vi "Host-Scannig-Probe-Microscope-Controller-2014-12-05-RFR-version-for-MCL-drift-trial-fm-NanoH50-1b.vi"() -> ()   [LabVIEW 2012]
uses:
  <vilib>/FPGAPlugInAG/PCIe-7852R/niLvFpga_Open_PCIe-7852R.vi
  <vilib>/Utility/error.llb/Error Cluster From Error Code.vi
  <vilib>/rvi/errors/niLvFpgaAdjustHostInterfaceError.vi
  <vilib>/FPGAPlugInAG/PCIe-7852R/niLvFpga_Close_PCIe-7852R.vi
  <vilib>/FPGAPlugInAG/PCIe-7852R/niLvFpga_Run_PCIe-7852R.vi
  <vilib>/Utility/file.llb/Write To Spreadsheet File (I64).vi
  <vilib>/rvi/interface/nirviOpenFPGA/nirviOpenFPGA.xnode
  FPGA Bitfiles/2012-10-30-PhD_FPGATarget_Scannig-Probe-Mi_wQHWF7AZtyE.lvbitx
  Scannig-Probe-Microscope-Controller-2010-03-08-RFR-version-for-MCL-nanoh50-1b.vi
  <vilib>/rvi/interface/nirviMethod/nirviMethod.xnode
  <vilib>/rvi/interface/nirviReadWriteControl/nirviReadWriteControl.xnode
  <vilib>/rvi/interface/nirviCloseFPGA/nirviCloseFPGA.xnode
  <vilib>/rvi/errors/niLvFpgaMergeErrorWithErrorCode.vi
  <vilib>/FPGAPlugInAG/PCIe-7852R/niLvFpga_ReadFifo_PCIe-7852R.vi
  NiFpgaLv.dll
panel:
  out "fpga y images":i32
  out "hi(x)":u16[](array[numeric])=[32260, 32260, 32276, 32269, 32267, 32261, 32276, 32257, 32271, 32261, 32259, 32255, 32261, 32255, 32257, 32259, 32264, 32267, 32261, 32276, 32252, 32274, 32264, 32263, 32267, 32260, 32257, 32262, 32260, 32263, 32265, 32252, 32248, 32257, 32271, 32258, 32258, 32267, 32259, 32260, 32276, 32276, 32254, 32257, 32255, 32263, 32266, 32260, 32264, 32256, 32262, 32259, 32264, 32267, 32255, 32256, 32271, 32257, 32260, 32265, 32260, 32258, 32277, 32257, 32267, 32253, 32260, 32257, 32262, 32264, 32264, 32263, 32260, 32266, 32254, 32263, 32261, 32256, 32269, 32265, 32263, 32279, 32265, 32262, 32253, 32269, 32266, 32269, 32257, 32262, 32249, 32260, 32251, 32259, 32265, 32264, 32262, 32261, 32259, 32268, 32260, 32260, 32277, 32271, 32242, 32256, 32253, 32257, 32257, 32237, 32263, 32250, 32261, 32264, 32273, 32263, 32258, 32264, 32259, 32265, 32256, 32263, 32264, 32277, 32271, 32255, 32258, 32261]
  out "Y line":i32=1
  out "Time per step (us) /X axis sub pixels":u32=203
  in  "X axis pixels":u16=256
  in  "Lines per second":dbl=0.2 min=1e-05 max=50.0
  in  "Time per step/ Y axis sub pixels (usec)":u32=1200
  in  "X Size (um)":dbl=60.0
  in  "X Total Range (um)":dbl=80.0
  in  "Y Size (um)":dbl=60.0
  in  "Y Total Range (um)":dbl=80.0
  in  "Y axis pixels":u16=256
  in  "Timeout FIFO":i32=-1
  in  "x initial":i16
  in  "y initial":i16
  out "X axis steps per pixel":u16=96
  in  "Number of images":u32=10000
  out "Y axis steps per pixel":u16=96
  out "Pixels for one image":i32=131072
  in  "Internal Setpoint":i16=7166
  in  "I scale":i8=-8
  in  "P scale":i8=-2
  in  "Setpoint Control":bool=TRUE
  in  "PID gains (x 2^8)":T1={"proportional gain (Kc)"=1, "integral gain (Kc*Ts/Ti)"=11, "derivative gain (Kc*Td/Ts)"=0}
  in  "Forth/Back X axis":bool
  in  "Forth/Back Y axis":bool
  in  "Feedback loop time(uSec)":u8
  in  "Stop Feedback":bool=TRUE
  in  "Scanning On/Off":bool
  in  "offset retraction drift":i16
  in  "control for drift correction":u32=512000
  in  "time before averaging drift":u32=9000
  in  "drift averager":u16=100
  in  "drift Waiting (uSec)":u16=10
  in  "offset FM":u16=1000
  out "Steps Per Feedback region":u16=642
  in  "Number of Feedback Regions":u32=102
  in  "shift integrator control":i32=2000
  in  "upper limit regions":i16=99
  out "line shift":i32
  out "line in matrix":i32=254
  out "Y Output Value":i16
  out "image indicator":i32=1
  out "Bottom Sensor Magnitude Image":i16[][](graph)
  out "Trace Bottom Sensor Magnitude":i16[][](graph)=[[12, 13, 14, 14, 14, 14, 14, 14, 14, 14, 14, 14, 14, 14, 14, 14, 14, 14, 14, 14, 14, 14, 14, 14, 14, 14, 14, 14, 14, 14, 14, 14, 14, 14, 14, 14, 14, 14, 14, 14, 14, 14, 14, 14, 14, 14, 14, 14, 14, 14, 14, 14, 14, 14, 14, 14, 14, 14, 14, 14, 14, 14, 14, 14, 14, 14, 14, 14, 14, 14, 14, 14, 14, 14, 14, 14, 14, 14, 14, 14, 14, 14, 14, 14, 14, 14, 14, 14, 14, 14, 14, 14, 14, 14, 14, 14, 14, 14, 14, 14, 14, 14, 14, 14, 14, 14, 14, 14, 14, 14, 14, 14, 14, 14, 14, 14, 14, 14, 14, 14, 14, 14, 14, 14, 14, 14, 14, 14, 14, 14, 14, 14, 14, 14, 14, 14, 14, 14, 14, 14, 14, 14, 14, 14, 14, 14, 14, 14, 14, 14, 14, 14, 14, 14, 14, 14, 14, 14, 14, 14, 14, 14, 14, 14, 14, 14, 14, 14, 14, 14, 14, 14, 14, 14, 14, 14, 14, 14, 14, 14, 14, 14, 14, 14, 14, 14, 14, 14, 14, 14, 14, 14, 14, 14, 14, 14, 14, 14, 14, 14, 14, 14, 14, 14, 14, 14, 14, 14, 14, 14, 14, 14, 14, 14, 14, 14, 14, 14, 14, 14, 14, 14, 14, 14, 14, 14, 14, 14, 14, 14, 14, 14, 14, 14, 14, 14, 14, 14, 14, 14, 14, 14, 14, 14, 14, 14, 14, 14, 14, 14, 14, 14, 14, 14, 14, 14], [10, 10, 10, 10, 11, 11, 11, 10, 10, 10, 10, 10, 10, 10, 10, 10, 10, 10, 10, 10, 10, 10, 10, 11, 11, 10, 10, 11, 11, 11, 11, 10, 10, 10, 10, 10, 10, 10, 10, 10, 11, 11, 10, 10, 11, 11, 11, 11, 11, 11, 10, 11, 11, 11, 11, 10, 10, 10, 10, 11, 10, 10, 10, 10, 10, 10, 10, 10, 10, 10, 11, 10, 10, 10, 10, 11, 11, 10, 10, 10, 10, 10, 10, 10, 10, 10, 10, 10, 10, 10, 10, 10, 10, 10, 10, 10, 10, 10, 10, 10, 10, 10, 10, 10, 10, 10, 10, 10, 10, 10, 11, 11, 10, 10, 10, 10, 11, 11, 11, 10, 10, 11, 10, 10, 10, 11, 11, 11, 11, 10, 10, 11, 11, 11, 10, 10, 11, 11, 10, 10, 10, 10, 10, 10, 10, 10, 11, 10, 10, 10, 10, 11, 11, 10, 10, 10, 10, 10, 10, 11, 11, 11, 11, 11, 11, 10, 10, 10, 10, 10, 10, 10, 10, 10, 10, 10, 10, 10, 10, 10, 10, 10, 10, 10, 11, 11, 10, 10, 10, 10, 10, 10, 11, 10, 10, 10, 11, 10, 10, 10, 10, 10, 10, 10, 10, 10, 10, 11, 11, 10, 10, 10, 11, 10, 10, 10, 10, 10, 10, 10, 10, 10, 11, 10, 10, 10, 10, 11, 11, 10, 10, 11, 11, 11, 11, 11, 11, 10, 10, 11, 11, 11, 11, 11, 11, 10, 10, 10, 10, 11, 10, 10, 10, 11, 13, 14]]
  out "TF Magnitude Image":i16[][](graph)
  out "Trace TF Magnitud":i16[][](graph)=[[18, 18, 18, 18, 18, 18, 18, 19, 19, 17, 17, 17, 18, 18, 18, 18, 18, 18, 18, 18, 18, 18, 18, 17, 17, 17, 17, 18, 18, 18, 17, 16, 16, 16, 16, 17, 18, 19, 20, 20, 19, 18, 18, 18, 18, 18, 18, 18, 17, 16, 16, 18, 19, 19, 18, 18, 18, 19, 20, 19, 18, 18, 18, 18, 18, 18, 18, 18, 18, 18, 17, 17, 17, 18, 18, 18, 18, 18, 18, 17, 17, 17, 18, 18, 18, 17, 16, 17, 17, 17, 17, 18, 18, 18, 17, 17, 18, 17, 17, 17, 17, 18, 18, 18, 18, 18, 18, 18, 17, 17, 18, 18, 18, 18, 18, 18, 18, 18, 19, 20, 19, 18, 16, 17, 18, 18, 17, 17, 17, 18, 18, 17, 17, 17, 16, 17, 18, 18, 18, 18, 18, 18, 18, 18, 17, 17, 17, 16, 16, 17, 18, 18, 18, 17, 17, 18, 19, 19, 18, 18, 18, 18, 17, 17, 18, 18, 18, 17, 17, 17, 17, 18, 18, 18, 18, 18, 17, 17, 17, 17, 17, 18, 18, 18, 18, 18, 18, 18, 18, 18, 18, 17, 16, 17, 17, 18, 19, 20, 19, 18, 18, 18, 18, 18, 17, 16, 16, 16, 16, 16, 16, 17, 18, 18, 17, 16, 17, 18, 18, 18, 18, 18, 17, 18, 18, 18, 18, 18, 18, 17, 17, 18, 18, 18, 18, 18, 18, 18, 18, 18, 19, 20, 19, 19, 18, 18, 18, 18, 17, 17, 17, 17, 18, 18, 18, 17], [17, 17, 17, 17, 17, 18, 18, 18, 18, 18, 18, 18, 17, 17, 17, 18, 18, 18, 19, 19, 19, 18, 18, 17, 18, 18, 18, 18, 18, 17, 18, 18, 19, 19, 18, 17, 17, 17, 17, 17, 17, 17, 17, 17, 17, 18, 18, 17, 17, 18, 19, 18, 17, 18, 18, 18, 18, 17, 17, 17, 18, 18, 18, 17, 16, 16, 17, 18, 19, 19, 18, 18, 19, 19, 18, 18, 18, 18, 17, 17, 16, 17, 18, 18, 18, 18, 18, 17, 17, 17, 18, 18, 18, 19, 18, 18, 17, 17, 17, 16, 16, 17, 16, 17, 18, 18, 18, 18, 18, 18, 18, 18, 18, 18, 18, 19, 20, 20, 19, 18, 18, 18, 18, 18, 19, 19, 18, 17, 17, 18, 18, 18, 18, 18, 18, 17, 18, 18, 18, 18, 17, 17, 17, 17, 18, 18, 18, 18, 18, 18, 17, 17, 17, 18, 18, 18, 18, 18, 18, 18, 18, 18, 18, 18, 18, 18, 18, 17, 17, 18, 18, 18, 18, 18, 18, 18, 18, 18, 18, 18, 18, 18, 18, 18, 17, 17, 18, 18, 18, 18, 17, 17, 17, 18, 18, 18, 18, 18, 18, 18, 18, 18, 18, 18, 18, 17, 16, 16, 16, 17, 18, 18, 18, 18, 17, 17, 17, 18, 18, 18, 17, 16, 17, 18, 18, 18, 18, 18, 18, 18, 18, 17, 16, 17, 18, 18, 18, 18, 18, 18, 18, 18, 18, 18, 18, 18, 18, 18, 17, 17, 18, 18, 18, 18, 18, 17]]
  out "Trace AI5 array":i16[][](array[numeric])=[[12, 13, 14, 14, 14, 14, 14, 14, 14, 14, 14, 14, 14, 14, 14, 14, 14, 14, 14, 14, 14, 14, 14, 14, 14, 14, 14, 14, 14, 14, 14, 14, 14, 14, 14, 14, 14, 14, 14, 14, 14, 14, 14, 14, 14, 14, 14, 14, 14, 14, 14, 14, 14, 14, 14, 14, 14, 14, 14, 14, 14, 14, 14, 14, 14, 14, 14, 14, 14, 14, 14, 14, 14, 14, 14, 14, 14, 14, 14, 14, 14, 14, 14, 14, 14, 14, 14, 14, 14, 14, 14, 14, 14, 14, 14, 14, 14, 14, 14, 14, 14, 14, 14, 14, 14, 14, 14, 14, 14, 14, 14, 14, 14, 14, 14, 14, 14, 14, 14, 14, 14, 14, 14, 14, 14, 14, 14, 14, 14, 14, 14, 14, 14, 14, 14, 14, 14, 14, 14, 14, 14, 14, 14, 14, 14, 14, 14, 14, 14, 14, 14, 14, 14, 14, 14, 14, 14, 14, 14, 14, 14, 14, 14, 14, 14, 14, 14, 14, 14, 14, 14, 14, 14, 14, 14, 14, 14, 14, 14, 14, 14, 14, 14, 14, 14, 14, 14, 14, 14, 14, 14, 14, 14, 14, 14, 14, 14, 14, 14, 14, 14, 14, 14, 14, 14, 14, 14, 14, 14, 14, 14, 14, 14, 14, 14, 14, 14, 14, 14, 14, 14, 14, 14, 14, 14, 14, 14, 14, 14, 14, 14, 14, 14, 14, 14, 14, 14, 14, 14, 14, 14, 14, 14, 14, 14, 14, 14, 14, 14, 14, 14, 14, 14, 14, 14, 14], [10, 10, 10, 10, 11, 11, 11, 10, 10, 10, 10, 10, 10, 10, 10, 10, 10, 10, 10, 10, 10, 10, 10, 11, 11, 10, 10, 11, 11, 11, 11, 10, 10, 10, 10, 10, 10, 10, 10, 10, 11, 11, 10, 10, 11, 11, 11, 11, 11, 11, 10, 11, 11, 11, 11, 10, 10, 10, 10, 11, 10, 10, 10, 10, 10, 10, 10, 10, 10, 10, 11, 10, 10, 10, 10, 11, 11, 10, 10, 10, 10, 10, 10, 10, 10, 10, 10, 10, 10, 10, 10, 10, 10, 10, 10, 10, 10, 10, 10, 10, 10, 10, 10, 10, 10, 10, 10, 10, 10, 10, 11, 11, 10, 10, 10, 10, 11, 11, 11, 10, 10, 11, 10, 10, 10, 11, 11, 11, 11, 10, 10, 11, 11, 11, 10, 10, 11, 11, 10, 10, 10, 10, 10, 10, 10, 10, 11, 10, 10, 10, 10, 11, 11, 10, 10, 10, 10, 10, 10, 11, 11, 11, 11, 11, 11, 10, 10, 10, 10, 10, 10, 10, 10, 10, 10, 10, 10, 10, 10, 10, 10, 10, 10, 10, 11, 11, 10, 10, 10, 10, 10, 10, 11, 10, 10, 10, 11, 10, 10, 10, 10, 10, 10, 10, 10, 10, 10, 11, 11, 10, 10, 10, 11, 10, 10, 10, 10, 10, 10, 10, 10, 10, 11, 10, 10, 10, 10, 11, 11, 10, 10, 11, 11, 11, 11, 11, 11, 10, 10, 11, 11, 11, 11, 11, 11, 10, 10, 10, 10, 11, 10, 10, 10, 11, 13, 14]]
  out "Trace AI5 temp":i16[](array[numeric])=[12, 13, 14, 14, 14, 14, 14, 14, 14, 14, 14, 14, 14, 14, 14, 14, 14, 14, 14, 14, 14, 14, 14, 14, 14, 14, 14, 14, 14, 14, 14, 14, 14, 14, 14, 14, 14, 14, 14, 14, 14, 14, 14, 14, 14, 14, 14, 14, 14, 14, 14, 14, 14, 14, 14, 14, 14, 14, 14, 14, 14, 14, 14, 14, 14, 14, 14, 14, 14, 14, 14, 14, 14, 14, 14, 14, 14, 14, 14, 14, 14, 14, 14, 14, 14, 14, 14, 14, 14, 14, 14, 14, 14, 14, 14, 14, 14, 14, 14, 14, 14, 14, 14, 14, 14, 14, 14, 14, 14, 14, 14, 14, 14, 14, 14, 14, 14, 14, 14, 14, 14, 14, 14, 14, 14, 14, 14, 14, 14, 14, 14, 14, 14, 14, 14, 14, 14, 14, 14, 14, 14, 14, 14, 14, 14, 14, 14, 14, 14, 14, 14, 14, 14, 14, 14, 14, 14, 14, 14, 14, 14, 14, 14, 14, 14, 14, 14, 14, 14, 14, 14, 14, 14, 14, 14, 14, 14, 14, 14, 14, 14, 14, 14, 14, 14, 14, 14, 14, 14, 14, 14, 14, 14, 14, 14, 14, 14, 14, 14, 14, 14, 14, 14, 14, 14, 14, 14, 14, 14, 14, 14, 14, 14, 14, 14, 14, 14, 14, 14, 14, 14, 14, 14, 14, 14, 14, 14, 14, 14, 14, 14, 14, 14, 14, 14, 14, 14, 14, 14, 14, 14, 14, 14, 14, 14, 14, 14, 14, 14, 14, 14, 14, 14, 14, 14, 14]
  out "Trace AI6  array":i16[][](array[numeric])=[[18, 18, 18, 18, 18, 18, 18, 19, 19, 17, 17, 17, 18, 18, 18, 18, 18, 18, 18, 18, 18, 18, 18, 17, 17, 17, 17, 18, 18, 18, 17, 16, 16, 16, 16, 17, 18, 19, 20, 20, 19, 18, 18, 18, 18, 18, 18, 18, 17, 16, 16, 18, 19, 19, 18, 18, 18, 19, 20, 19, 18, 18, 18, 18, 18, 18, 18, 18, 18, 18, 17, 17, 17, 18, 18, 18, 18, 18, 18, 17, 17, 17, 18, 18, 18, 17, 16, 17, 17, 17, 17, 18, 18, 18, 17, 17, 18, 17, 17, 17, 17, 18, 18, 18, 18, 18, 18, 18, 17, 17, 18, 18, 18, 18, 18, 18, 18, 18, 19, 20, 19, 18, 16, 17, 18, 18, 17, 17, 17, 18, 18, 17, 17, 17, 16, 17, 18, 18, 18, 18, 18, 18, 18, 18, 17, 17, 17, 16, 16, 17, 18, 18, 18, 17, 17, 18, 19, 19, 18, 18, 18, 18, 17, 17, 18, 18, 18, 17, 17, 17, 17, 18, 18, 18, 18, 18, 17, 17, 17, 17, 17, 18, 18, 18, 18, 18, 18, 18, 18, 18, 18, 17, 16, 17, 17, 18, 19, 20, 19, 18, 18, 18, 18, 18, 17, 16, 16, 16, 16, 16, 16, 17, 18, 18, 17, 16, 17, 18, 18, 18, 18, 18, 17, 18, 18, 18, 18, 18, 18, 17, 17, 18, 18, 18, 18, 18, 18, 18, 18, 18, 19, 20, 19, 19, 18, 18, 18, 18, 17, 17, 17, 17, 18, 18, 18, 17], [17, 17, 17, 17, 17, 18, 18, 18, 18, 18, 18, 18, 17, 17, 17, 18, 18, 18, 19, 19, 19, 18, 18, 17, 18, 18, 18, 18, 18, 17, 18, 18, 19, 19, 18, 17, 17, 17, 17, 17, 17, 17, 17, 17, 17, 18, 18, 17, 17, 18, 19, 18, 17, 18, 18, 18, 18, 17, 17, 17, 18, 18, 18, 17, 16, 16, 17, 18, 19, 19, 18, 18, 19, 19, 18, 18, 18, 18, 17, 17, 16, 17, 18, 18, 18, 18, 18, 17, 17, 17, 18, 18, 18, 19, 18, 18, 17, 17, 17, 16, 16, 17, 16, 17, 18, 18, 18, 18, 18, 18, 18, 18, 18, 18, 18, 19, 20, 20, 19, 18, 18, 18, 18, 18, 19, 19, 18, 17, 17, 18, 18, 18, 18, 18, 18, 17, 18, 18, 18, 18, 17, 17, 17, 17, 18, 18, 18, 18, 18, 18, 17, 17, 17, 18, 18, 18, 18, 18, 18, 18, 18, 18, 18, 18, 18, 18, 18, 17, 17, 18, 18, 18, 18, 18, 18, 18, 18, 18, 18, 18, 18, 18, 18, 18, 17, 17, 18, 18, 18, 18, 17, 17, 17, 18, 18, 18, 18, 18, 18, 18, 18, 18, 18, 18, 18, 17, 16, 16, 16, 17, 18, 18, 18, 18, 17, 17, 17, 18, 18, 18, 17, 16, 17, 18, 18, 18, 18, 18, 18, 18, 18, 17, 16, 17, 18, 18, 18, 18, 18, 18, 18, 18, 18, 18, 18, 18, 18, 18, 17, 17, 18, 18, 18, 18, 18, 17]]
  out "TraceAI6 temp":i16[](array[numeric])=[18, 18, 18, 18, 18, 18, 18, 19, 19, 17, 17, 17, 18, 18, 18, 18, 18, 18, 18, 18, 18, 18, 18, 17, 17, 17, 17, 18, 18, 18, 17, 16, 16, 16, 16, 17, 18, 19, 20, 20, 19, 18, 18, 18, 18, 18, 18, 18, 17, 16, 16, 18, 19, 19, 18, 18, 18, 19, 20, 19, 18, 18, 18, 18, 18, 18, 18, 18, 18, 18, 17, 17, 17, 18, 18, 18, 18, 18, 18, 17, 17, 17, 18, 18, 18, 17, 16, 17, 17, 17, 17, 18, 18, 18, 17, 17, 18, 17, 17, 17, 17, 18, 18, 18, 18, 18, 18, 18, 17, 17, 18, 18, 18, 18, 18, 18, 18, 18, 19, 20, 19, 18, 16, 17, 18, 18, 17, 17, 17, 18, 18, 17, 17, 17, 16, 17, 18, 18, 18, 18, 18, 18, 18, 18, 17, 17, 17, 16, 16, 17, 18, 18, 18, 17, 17, 18, 19, 19, 18, 18, 18, 18, 17, 17, 18, 18, 18, 17, 17, 17, 17, 18, 18, 18, 18, 18, 17, 17, 17, 17, 17, 18, 18, 18, 18, 18, 18, 18, 18, 18, 18, 17, 16, 17, 17, 18, 19, 20, 19, 18, 18, 18, 18, 18, 17, 16, 16, 16, 16, 16, 16, 17, 18, 18, 17, 16, 17, 18, 18, 18, 18, 18, 17, 18, 18, 18, 18, 18, 18, 17, 17, 18, 18, 18, 18, 18, 18, 18, 18, 18, 19, 20, 19, 19, 18, 18, 18, 18, 17, 17, 17, 17, 18, 18, 18, 17]
  out "AI5 Back":i16[][](array[numeric])
  out "AI5 Array":i16[][](array[numeric])
  out "AI6 Array Back":i16[][](array[numeric])
  out "AI6 Array":i16[][](array[numeric])
  out "Internal Setpoint indicator":i16=7166
  out "iterations x":i32=1023
  out "Trace AI2 array":i16[][](array[numeric])=[[32261, 32262, 32263, 32251, 32270, 32257, 32263, 32257, 32274, 32262, 32258, 32261, 32254, 32263, 32267, 32265, 32263, 32260, 32249, 32260, 32251, 32264, 32255, 32260, 32266, 32263, 32269, 32248, 32264, 32262, 32268, 32250, 32269, 32263, 32260, 32264, 32263, 32260, 32236, 32261, 32253, 32255, 32266, 32261, 32263, 32258, 32276, 32246, 32255, 32242, 32251, 32252, 32264, 32263, 32258, 32254, 32261, 32247, 32260, 32251, 32249, 32263, 32256, 32251, 32273, 32242, 32249, 32257, 32259, 32262, 32260, 32251, 32264, 32260, 32267, 32257, 32267, 32257, 32270, 32255, 32253, 32261, 32258, 32264, 32261, 32261, 32259, 32266, 32261, 32255, 32254, 32243, 32258, 32270, 32261, 32268, 32265, 32260, 32259, 32262, 32263, 32248, 32261, 32261, 32264, 32283, 32264, 32255, 32252, 32251, 32266, 32260, 32258, 32258, 32261, 32256, 32262, 32256, 32281, 32258, 32262, 32255, 32267, 32263, 32274, 32255, 32261, 32261, 32264, 32261, 32264, 32256, 32266, 32276, 32254, 32267, 32263, 32252, 32261, 32275, 32279, 32262, 32254, 32263, 32265, 32261, 32270, 32270, 32256, 32261, 32264, 32265, 32246, 32257, 32259, 32259, 32257, 32259, 32270, 32265, 32263, 32262, 32241, 32262, 32263, 32263, 32252, 32264, 32260, 32270, 32260, 32258, 32261, 32258, 32268, 32269, 32272, 32261, 32249, 32278, 32265, 32259, 32250, 32254, 32267, 32264, 32261, 32255, 32259, 32257, 32264, 32258, 32261, 32259, 32247, 32249, 32263, 32255, 32264, 32253, 32258, 32259, 32261, 32262, 32262, 32264, 32257, 32270, 32274, 32264, 32275, 32260, 32266, 32269, 32250, 32258, 32254, 32260, 32255, 32265, 32269, 32271, 32264, 32257, 32260, 32259, 32239, 32242, 32255, 32263, 32257, 32263, 32258, 32255, 32259, 32259, 32255, 32271, 32258, 32250, 32265, 32249, 32257, 32258, 32265, 32264, 32261, 32259, 32263, 32265, 32259, 32267, 32258, 32251, 32265, 32258], [32256, 32261, 32264, 32269, 32254, 32261, 32261, 32260, 32262, 32261, 32264, 32263, 32264, 32247, 32264, 32256, 32262, 32263, 32258, 32274, 32252, 32260, 32259, 32255, 32266, 32259, 32252, 32258, 32279, 32246, 32265, 32261, 32259, 32259, 32260, 32265, 32248, 32273, 32261, 32246, 32261, 32261, 32266, 32248, 32258, 32262, 32269, 32242, 32261, 32261, 32264, 32263, 32258, 32262, 32240, 32263, 32254, 32266, 32258, 32266, 32259, 32251, 32250, 32257, 32262, 32259, 32260, 32263, 32261, 32251, 32259, 32269, 32263, 32261, 32262, 32260, 32256, 32260, 32262, 32257, 32259, 32263, 32260, 32261, 32263, 32259, 32257, 32258, 32256, 32277, 32264, 32260, 32254, 32264, 32269, 32259, 32261, 32249, 32256, 32260, 32258, 32252, 32261, 32258, 32259, 32267, 32252, 32261, 32269, 32256, 32235, 32265, 32252, 32256, 32263, 32261, 32266, 32255, 32246, 32261, 32255, 32261, 32263, 32261, 32259, 32258, 32248, 32266, 32261, 32258, 32255, 32271, 32277, 32264, 32263, 32256, 32265, 32259, 32264, 32258, 32263, 32273, 32264, 32261, 32250, 32263, 32237, 32257, 32257, 32253, 32256, 32242, 32271, 32277, 32260, 32260, 32268, 32259, 32261, 32262, 32264, 32265, 32259, 32251, 32260, 32249, 32262, 32257, 32269, 32266, 32269, 32253, 32262, 32265, 32279, 32263, 32265, 32269, 32256, 32261, 32263, 32254, 32266, 32260, 32263, 32264, 32264, 32262, 32257, 32260, 32253, 32267, 32257, 32277, 32258, 32260, 32265, 32260, 32257, 32271, 32256, 32255, 32267, 32264, 32259, 32262, 32256, 32264, 32260, 32266, 32263, 32255, 32257, 32254, 32276, 32276, 32260, 32259, 32267, 32258, 32258, 32271, 32257, 32248, 32252, 32265, 32263, 32260, 32262, 32257, 32260, 32267, 32263, 32264, 32274, 32252, 32276, 32261, 32267, 32264, 32259, 32257, 32255, 32261, 32255, 32259, 32261, 32271, 32257, 32276, 32261, 32267, 32269, 32276, 32260, 32260]]
  out "TraceAI2 array temp":i16[](array[numeric])=[32261, 32262, 32263, 32251, 32270, 32257, 32263, 32257, 32274, 32262, 32258, 32261, 32254, 32263, 32267, 32265, 32263, 32260, 32249, 32260, 32251, 32264, 32255, 32260, 32266, 32263, 32269, 32248, 32264, 32262, 32268, 32250, 32269, 32263, 32260, 32264, 32263, 32260, 32236, 32261, 32253, 32255, 32266, 32261, 32263, 32258, 32276, 32246, 32255, 32242, 32251, 32252, 32264, 32263, 32258, 32254, 32261, 32247, 32260, 32251, 32249, 32263, 32256, 32251, 32273, 32242, 32249, 32257, 32259, 32262, 32260, 32251, 32264, 32260, 32267, 32257, 32267, 32257, 32270, 32255, 32253, 32261, 32258, 32264, 32261, 32261, 32259, 32266, 32261, 32255, 32254, 32243, 32258, 32270, 32261, 32268, 32265, 32260, 32259, 32262, 32263, 32248, 32261, 32261, 32264, 32283, 32264, 32255, 32252, 32251, 32266, 32260, 32258, 32258, 32261, 32256, 32262, 32256, 32281, 32258, 32262, 32255, 32267, 32263, 32274, 32255, 32261, 32261, 32264, 32261, 32264, 32256, 32266, 32276, 32254, 32267, 32263, 32252, 32261, 32275, 32279, 32262, 32254, 32263, 32265, 32261, 32270, 32270, 32256, 32261, 32264, 32265, 32246, 32257, 32259, 32259, 32257, 32259, 32270, 32265, 32263, 32262, 32241, 32262, 32263, 32263, 32252, 32264, 32260, 32270, 32260, 32258, 32261, 32258, 32268, 32269, 32272, 32261, 32249, 32278, 32265, 32259, 32250, 32254, 32267, 32264, 32261, 32255, 32259, 32257, 32264, 32258, 32261, 32259, 32247, 32249, 32263, 32255, 32264, 32253, 32258, 32259, 32261, 32262, 32262, 32264, 32257, 32270, 32274, 32264, 32275, 32260, 32266, 32269, 32250, 32258, 32254, 32260, 32255, 32265, 32269, 32271, 32264, 32257, 32260, 32259, 32239, 32242, 32255, 32263, 32257, 32263, 32258, 32255, 32259, 32259, 32255, 32271, 32258, 32250, 32265, 32249, 32257, 32258, 32265, 32264, 32261, 32259, 32263, 32265, 32259, 32267, 32258, 32251, 32265, 32258]
  out "Trace Topography Array":i32[][](array[numeric])
  out "Trace Topography Array temp":i32[](array[numeric])
  out "Trace AI0 Array":i16[][](array[numeric])=[[11115, 11122, 11110, 11108, 11107, 11109, 11113, 11126, 11120, 11117, 11099, 11120, 11114, 11107, 11113, 11109, 11112, 11105, 11118, 11111, 11122, 11105, 11114, 11116, 11108, 11103, 11125, 11106, 11108, 11089, 11098, 11100, 11098, 11128, 11115, 11109, 11115, 11129, 11126, 11102, 11107, 11104, 11120, 11112, 11110, 11122, 11096, 11111, 11101, 11125, 11117, 11119, 11118, 11120, 11103, 11103, 11093, 11103, 11112, 11096, 11092, 11117, 11106, 11103, 11079, 11113, 11102, 11116, 11113, 11106, 11108, 11115, 11118, 11092, 11103, 11108, 11108, 11097, 11130, 11112, 11097, 11091, 11085, 11102, 11115, 11104, 11103, 11107, 11123, 11117, 11120, 11104, 11109, 11107, 11102, 11110, 11091, 11107, 11117, 11107, 11097, 11098, 11118, 11097, 11128, 11080, 11107, 11099, 11121, 11097, 11111, 11123, 11108, 11122, 11111, 11113, 11127, 11113, 11096, 11108, 11103, 11123, 11106, 11109, 11105, 11110, 11091, 11104, 11109, 11104, 11103, 11106, 11093, 11113, 11101, 11094, 11095, 11092, 11093, 11107, 11111, 11106, 11105, 11102, 11095, 11120, 11094, 11101, 11117, 11109, 11091, 11107, 11108, 11116, 11128, 11092, 11111, 11105, 11102, 11089, 11096, 11097, 11109, 11114, 11118, 11128, 11116, 11106, 11109, 11095, 11100, 11110, 11122, 11103, 11099, 11106, 11086, 11116, 11100, 11091, 11115, 11103, 11106, 11100, 11104, 11126, 11112, 11111, 11102, 11096, 11090, 11110, 11093, 11100, 11108, 11119, 11101, 11112, 11095, 11111, 11105, 11116, 11101, 11104, 11104, 11094, 11105, 11106, 11110, 11101, 11112, 11098, 11105, 11118, 11112, 11103, 11109, 11116, 11110, 11113, 11112, 11109, 11109, 11121, 11104, 11104, 11105, 11113, 11107, 11100, 11117, 11124, 11114, 11095, 11088, 11102, 11113, 11113, 11111, 11107, 11105, 11111, 11096, 11079, 11119, 11104, 11094, 11093, 11129, 11125, 11082, 11093, 11120, 11096, 11103, 11112], [11110, 11097, 11117, 11109, 11114, 11108, 11110, 11119, 11110, 11092, 11106, 11121, 11101, 11105, 11130, 11108, 11093, 11111, 11105, 11106, 11111, 11122, 11115, 11087, 11103, 11110, 11108, 11093, 11105, 11101, 11111, 11112, 11101, 11117, 11107, 11125, 11115, 11106, 11107, 11100, 11121, 11105, 11106, 11112, 11083, 11110, 11102, 11093, 11107, 11128, 11107, 11121, 11118, 11108, 11123, 11099, 11115, 11101, 11099, 11111, 11119, 11111, 11108, 11115, 11115, 11113, 11102, 11103, 11123, 11120, 11109, 11091, 11099, 11101, 11101, 11096, 11105, 11097, 11099, 11111, 11102, 11098, 11104, 11099, 11122, 11120, 11121, 11102, 11099, 11094, 11106, 11115, 11096, 11113, 11107, 11109, 11116, 11107, 11126, 11103, 11113, 11111, 11098, 11104, 11108, 11121, 11114, 11102, 11118, 11117, 11130, 11114, 11116, 11101, 11106, 11106, 11108, 11100, 11113, 11102, 11110, 11108, 11097, 11087, 11109, 11105, 11114, 11090, 11108, 11094, 11100, 11097, 11117, 11094, 11111, 11113, 11109, 11108, 11115, 11112, 11109, 11095, 11111, 11091, 11098, 11122, 11110, 11112, 11126, 11086, 11103, 11105, 11094, 11107, 11100, 11128, 11103, 11113, 11109, 11099, 11096, 11086, 11101, 11109, 11118, 11109, 11100, 11090, 11089, 11105, 11104, 11109, 11103, 11094, 11105, 11105, 11107, 11104, 11105, 11111, 11113, 11107, 11112, 11110, 11101, 11113, 11112, 11099, 11087, 11086, 11103, 11115, 11110, 11114, 11106, 11118, 11111, 11111, 11109, 11119, 11102, 11111, 11094, 11105, 11113, 11122, 11124, 11112, 11121, 11113, 11111, 11130, 11111, 11107, 11095, 11129, 11110, 11113, 11126, 11099, 11105, 11101, 11090, 11132, 11125, 11098, 11105, 11102, 11102, 11099, 11107, 11105, 11112, 11127, 11124, 11103, 11105, 11098, 11098, 11100, 11115, 11100, 11118, 11103, 11107, 11098, 11105, 11100, 11093, 11089, 11099, 11101, 11083, 11115, 11103, 11097]]
  out "Trace AI0 array temp":i16[](array[numeric])=[11115, 11122, 11110, 11108, 11107, 11109, 11113, 11126, 11120, 11117, 11099, 11120, 11114, 11107, 11113, 11109, 11112, 11105, 11118, 11111, 11122, 11105, 11114, 11116, 11108, 11103, 11125, 11106, 11108, 11089, 11098, 11100, 11098, 11128, 11115, 11109, 11115, 11129, 11126, 11102, 11107, 11104, 11120, 11112, 11110, 11122, 11096, 11111, 11101, 11125, 11117, 11119, 11118, 11120, 11103, 11103, 11093, 11103, 11112, 11096, 11092, 11117, 11106, 11103, 11079, 11113, 11102, 11116, 11113, 11106, 11108, 11115, 11118, 11092, 11103, 11108, 11108, 11097, 11130, 11112, 11097, 11091, 11085, 11102, 11115, 11104, 11103, 11107, 11123, 11117, 11120, 11104, 11109, 11107, 11102, 11110, 11091, 11107, 11117, 11107, 11097, 11098, 11118, 11097, 11128, 11080, 11107, 11099, 11121, 11097, 11111, 11123, 11108, 11122, 11111, 11113, 11127, 11113, 11096, 11108, 11103, 11123, 11106, 11109, 11105, 11110, 11091, 11104, 11109, 11104, 11103, 11106, 11093, 11113, 11101, 11094, 11095, 11092, 11093, 11107, 11111, 11106, 11105, 11102, 11095, 11120, 11094, 11101, 11117, 11109, 11091, 11107, 11108, 11116, 11128, 11092, 11111, 11105, 11102, 11089, 11096, 11097, 11109, 11114, 11118, 11128, 11116, 11106, 11109, 11095, 11100, 11110, 11122, 11103, 11099, 11106, 11086, 11116, 11100, 11091, 11115, 11103, 11106, 11100, 11104, 11126, 11112, 11111, 11102, 11096, 11090, 11110, 11093, 11100, 11108, 11119, 11101, 11112, 11095, 11111, 11105, 11116, 11101, 11104, 11104, 11094, 11105, 11106, 11110, 11101, 11112, 11098, 11105, 11118, 11112, 11103, 11109, 11116, 11110, 11113, 11112, 11109, 11109, 11121, 11104, 11104, 11105, 11113, 11107, 11100, 11117, 11124, 11114, 11095, 11088, 11102, 11113, 11113, 11111, 11107, 11105, 11111, 11096, 11079, 11119, 11104, 11094, 11093, 11129, 11125, 11082, 11093, 11120, 11096, 11103, 11112]
  out "X Output Value":i16
  out "AI2 Array back":i16[][](array[numeric])
  out "AI0 back":i16[][](array[numeric])
  out "Topography Array back":i32[][](array[numeric])
  out "Command Out":i16
  out "counter":i16
  in  "Topo Prefix 2":string
  in  "Topo Prefix 1":string
  in  "Phase Prefix 2":string
  in  "Phase Prefix 1":string
  in  "Freq Prefix 2":string
  in  "Freq Prefix 1":string
  in  "Data Directory":path=path "C:/Users/Rodolfo/Documents/LAB/2013-02-24-SPM-data"
  out "Inidicator  forth/back  Y axis":i8=1
  out "Topography Image":i32[][](graph)
  out "Trace  Topography":i32[][](graph)
  out "Topography Array":i32[][](array[numeric])
  in  "New Image":bool
  out "error out 2":errorcluster
  out "error out":errorcluster
  out "Bottom Sensor Phase  Image":i16[][](graph)
  out "Trace Bottom Sensor Phase":i16[][](graph)=[[11115, 11122, 11110, 11108, 11107, 11109, 11113, 11126, 11120, 11117, 11099, 11120, 11114, 11107, 11113, 11109, 11112, 11105, 11118, 11111, 11122, 11105, 11114, 11116, 11108, 11103, 11125, 11106, 11108, 11089, 11098, 11100, 11098, 11128, 11115, 11109, 11115, 11129, 11126, 11102, 11107, 11104, 11120, 11112, 11110, 11122, 11096, 11111, 11101, 11125, 11117, 11119, 11118, 11120, 11103, 11103, 11093, 11103, 11112, 11096, 11092, 11117, 11106, 11103, 11079, 11113, 11102, 11116, 11113, 11106, 11108, 11115, 11118, 11092, 11103, 11108, 11108, 11097, 11130, 11112, 11097, 11091, 11085, 11102, 11115, 11104, 11103, 11107, 11123, 11117, 11120, 11104, 11109, 11107, 11102, 11110, 11091, 11107, 11117, 11107, 11097, 11098, 11118, 11097, 11128, 11080, 11107, 11099, 11121, 11097, 11111, 11123, 11108, 11122, 11111, 11113, 11127, 11113, 11096, 11108, 11103, 11123, 11106, 11109, 11105, 11110, 11091, 11104, 11109, 11104, 11103, 11106, 11093, 11113, 11101, 11094, 11095, 11092, 11093, 11107, 11111, 11106, 11105, 11102, 11095, 11120, 11094, 11101, 11117, 11109, 11091, 11107, 11108, 11116, 11128, 11092, 11111, 11105, 11102, 11089, 11096, 11097, 11109, 11114, 11118, 11128, 11116, 11106, 11109, 11095, 11100, 11110, 11122, 11103, 11099, 11106, 11086, 11116, 11100, 11091, 11115, 11103, 11106, 11100, 11104, 11126, 11112, 11111, 11102, 11096, 11090, 11110, 11093, 11100, 11108, 11119, 11101, 11112, 11095, 11111, 11105, 11116, 11101, 11104, 11104, 11094, 11105, 11106, 11110, 11101, 11112, 11098, 11105, 11118, 11112, 11103, 11109, 11116, 11110, 11113, 11112, 11109, 11109, 11121, 11104, 11104, 11105, 11113, 11107, 11100, 11117, 11124, 11114, 11095, 11088, 11102, 11113, 11113, 11111, 11107, 11105, 11111, 11096, 11079, 11119, 11104, 11094, 11093, 11129, 11125, 11082, 11093, 11120, 11096, 11103, 11112], [11110, 11097, 11117, 11109, 11114, 11108, 11110, 11119, 11110, 11092, 11106, 11121, 11101, 11105, 11130, 11108, 11093, 11111, 11105, 11106, 11111, 11122, 11115, 11087, 11103, 11110, 11108, 11093, 11105, 11101, 11111, 11112, 11101, 11117, 11107, 11125, 11115, 11106, 11107, 11100, 11121, 11105, 11106, 11112, 11083, 11110, 11102, 11093, 11107, 11128, 11107, 11121, 11118, 11108, 11123, 11099, 11115, 11101, 11099, 11111, 11119, 11111, 11108, 11115, 11115, 11113, 11102, 11103, 11123, 11120, 11109, 11091, 11099, 11101, 11101, 11096, 11105, 11097, 11099, 11111, 11102, 11098, 11104, 11099, 11122, 11120, 11121, 11102, 11099, 11094, 11106, 11115, 11096, 11113, 11107, 11109, 11116, 11107, 11126, 11103, 11113, 11111, 11098, 11104, 11108, 11121, 11114, 11102, 11118, 11117, 11130, 11114, 11116, 11101, 11106, 11106, 11108, 11100, 11113, 11102, 11110, 11108, 11097, 11087, 11109, 11105, 11114, 11090, 11108, 11094, 11100, 11097, 11117, 11094, 11111, 11113, 11109, 11108, 11115, 11112, 11109, 11095, 11111, 11091, 11098, 11122, 11110, 11112, 11126, 11086, 11103, 11105, 11094, 11107, 11100, 11128, 11103, 11113, 11109, 11099, 11096, 11086, 11101, 11109, 11118, 11109, 11100, 11090, 11089, 11105, 11104, 11109, 11103, 11094, 11105, 11105, 11107, 11104, 11105, 11111, 11113, 11107, 11112, 11110, 11101, 11113, 11112, 11099, 11087, 11086, 11103, 11115, 11110, 11114, 11106, 11118, 11111, 11111, 11109, 11119, 11102, 11111, 11094, 11105, 11113, 11122, 11124, 11112, 11121, 11113, 11111, 11130, 11111, 11107, 11095, 11129, 11110, 11113, 11126, 11099, 11105, 11101, 11090, 11132, 11125, 11098, 11105, 11102, 11102, 11099, 11107, 11105, 11112, 11127, 11124, 11103, 11105, 11098, 11098, 11100, 11115, 11100, 11118, 11103, 11107, 11098, 11105, 11100, 11093, 11089, 11099, 11101, 11083, 11115, 11103, 11097]]
  out "Trace Frequency":i16[][](graph)=[[32261, 32262, 32263, 32251, 32270, 32257, 32263, 32257, 32274, 32262, 32258, 32261, 32254, 32263, 32267, 32265, 32263, 32260, 32249, 32260, 32251, 32264, 32255, 32260, 32266, 32263, 32269, 32248, 32264, 32262, 32268, 32250, 32269, 32263, 32260, 32264, 32263, 32260, 32236, 32261, 32253, 32255, 32266, 32261, 32263, 32258, 32276, 32246, 32255, 32242, 32251, 32252, 32264, 32263, 32258, 32254, 32261, 32247, 32260, 32251, 32249, 32263, 32256, 32251, 32273, 32242, 32249, 32257, 32259, 32262, 32260, 32251, 32264, 32260, 32267, 32257, 32267, 32257, 32270, 32255, 32253, 32261, 32258, 32264, 32261, 32261, 32259, 32266, 32261, 32255, 32254, 32243, 32258, 32270, 32261, 32268, 32265, 32260, 32259, 32262, 32263, 32248, 32261, 32261, 32264, 32283, 32264, 32255, 32252, 32251, 32266, 32260, 32258, 32258, 32261, 32256, 32262, 32256, 32281, 32258, 32262, 32255, 32267, 32263, 32274, 32255, 32261, 32261, 32264, 32261, 32264, 32256, 32266, 32276, 32254, 32267, 32263, 32252, 32261, 32275, 32279, 32262, 32254, 32263, 32265, 32261, 32270, 32270, 32256, 32261, 32264, 32265, 32246, 32257, 32259, 32259, 32257, 32259, 32270, 32265, 32263, 32262, 32241, 32262, 32263, 32263, 32252, 32264, 32260, 32270, 32260, 32258, 32261, 32258, 32268, 32269, 32272, 32261, 32249, 32278, 32265, 32259, 32250, 32254, 32267, 32264, 32261, 32255, 32259, 32257, 32264, 32258, 32261, 32259, 32247, 32249, 32263, 32255, 32264, 32253, 32258, 32259, 32261, 32262, 32262, 32264, 32257, 32270, 32274, 32264, 32275, 32260, 32266, 32269, 32250, 32258, 32254, 32260, 32255, 32265, 32269, 32271, 32264, 32257, 32260, 32259, 32239, 32242, 32255, 32263, 32257, 32263, 32258, 32255, 32259, 32259, 32255, 32271, 32258, 32250, 32265, 32249, 32257, 32258, 32265, 32264, 32261, 32259, 32263, 32265, 32259, 32267, 32258, 32251, 32265, 32258], [32256, 32261, 32264, 32269, 32254, 32261, 32261, 32260, 32262, 32261, 32264, 32263, 32264, 32247, 32264, 32256, 32262, 32263, 32258, 32274, 32252, 32260, 32259, 32255, 32266, 32259, 32252, 32258, 32279, 32246, 32265, 32261, 32259, 32259, 32260, 32265, 32248, 32273, 32261, 32246, 32261, 32261, 32266, 32248, 32258, 32262, 32269, 32242, 32261, 32261, 32264, 32263, 32258, 32262, 32240, 32263, 32254, 32266, 32258, 32266, 32259, 32251, 32250, 32257, 32262, 32259, 32260, 32263, 32261, 32251, 32259, 32269, 32263, 32261, 32262, 32260, 32256, 32260, 32262, 32257, 32259, 32263, 32260, 32261, 32263, 32259, 32257, 32258, 32256, 32277, 32264, 32260, 32254, 32264, 32269, 32259, 32261, 32249, 32256, 32260, 32258, 32252, 32261, 32258, 32259, 32267, 32252, 32261, 32269, 32256, 32235, 32265, 32252, 32256, 32263, 32261, 32266, 32255, 32246, 32261, 32255, 32261, 32263, 32261, 32259, 32258, 32248, 32266, 32261, 32258, 32255, 32271, 32277, 32264, 32263, 32256, 32265, 32259, 32264, 32258, 32263, 32273, 32264, 32261, 32250, 32263, 32237, 32257, 32257, 32253, 32256, 32242, 32271, 32277, 32260, 32260, 32268, 32259, 32261, 32262, 32264, 32265, 32259, 32251, 32260, 32249, 32262, 32257, 32269, 32266, 32269, 32253, 32262, 32265, 32279, 32263, 32265, 32269, 32256, 32261, 32263, 32254, 32266, 32260, 32263, 32264, 32264, 32262, 32257, 32260, 32253, 32267, 32257, 32277, 32258, 32260, 32265, 32260, 32257, 32271, 32256, 32255, 32267, 32264, 32259, 32262, 32256, 32264, 32260, 32266, 32263, 32255, 32257, 32254, 32276, 32276, 32260, 32259, 32267, 32258, 32258, 32271, 32257, 32248, 32252, 32265, 32263, 32260, 32262, 32257, 32260, 32267, 32263, 32264, 32274, 32252, 32276, 32261, 32267, 32264, 32259, 32257, 32255, 32261, 32255, 32259, 32261, 32271, 32257, 32276, 32261, 32267, 32269, 32276, 32260, 32260]]
  out "Frequency Shift Image":i16[][](graph)
  out "AI0 Array":i16[][](array[numeric])
  out "AI2 Array":i16[][](array[numeric])
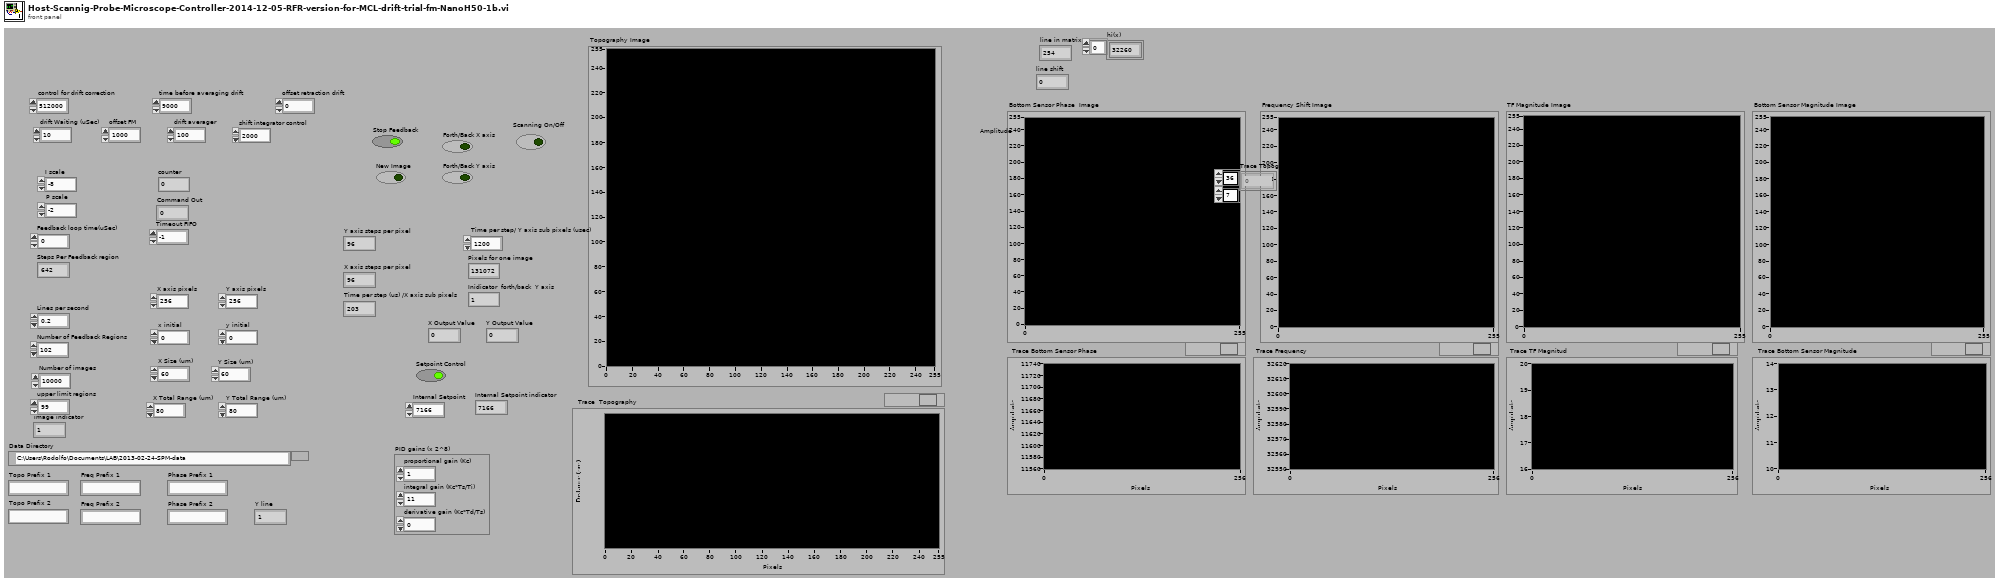
[diagram p1: front panel]
types:
  T1 = cluster{"proportional gain (Kc)":i16, "integral gain (Kc*Ts/Ti)":i16, "derivative gain (Kc*Td/Ts)":i16}
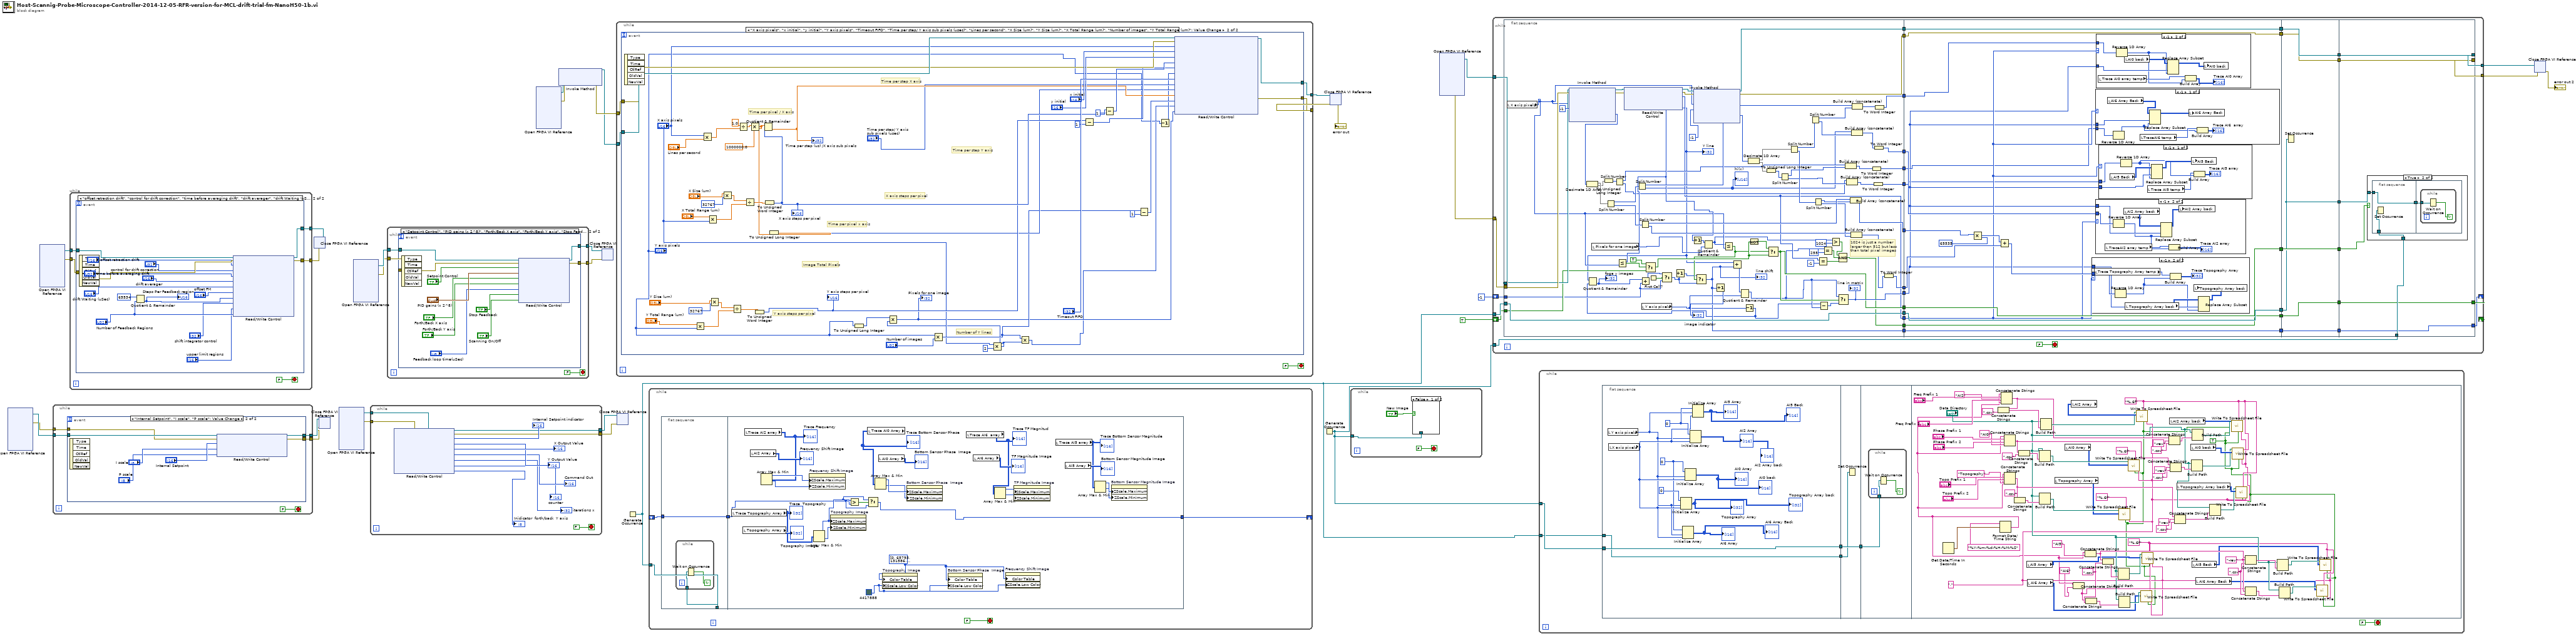
[diagram p0: block diagram]
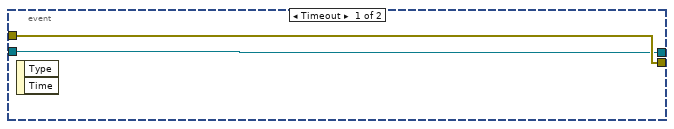
[diagram p2: hidden frame]
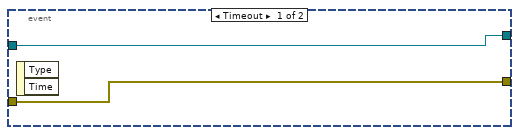
[diagram p3: hidden frame]
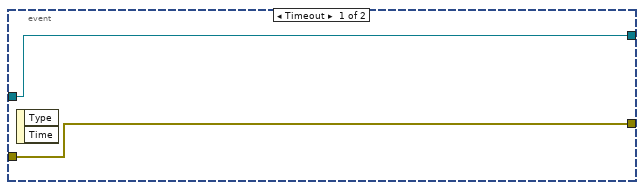
[diagram p4: hidden frame]
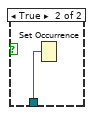
[diagram p5: hidden frame]
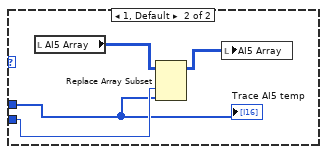
[diagram p6: hidden frame]
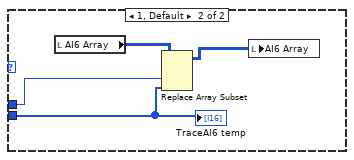
[diagram p7: hidden frame]
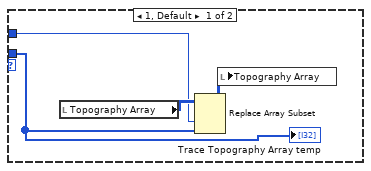
[diagram p8: hidden frame]
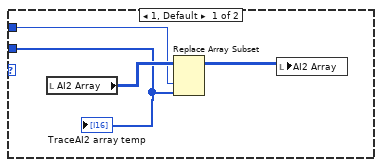
[diagram p9: hidden frame]
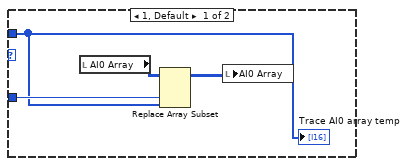
[diagram p10: hidden frame]
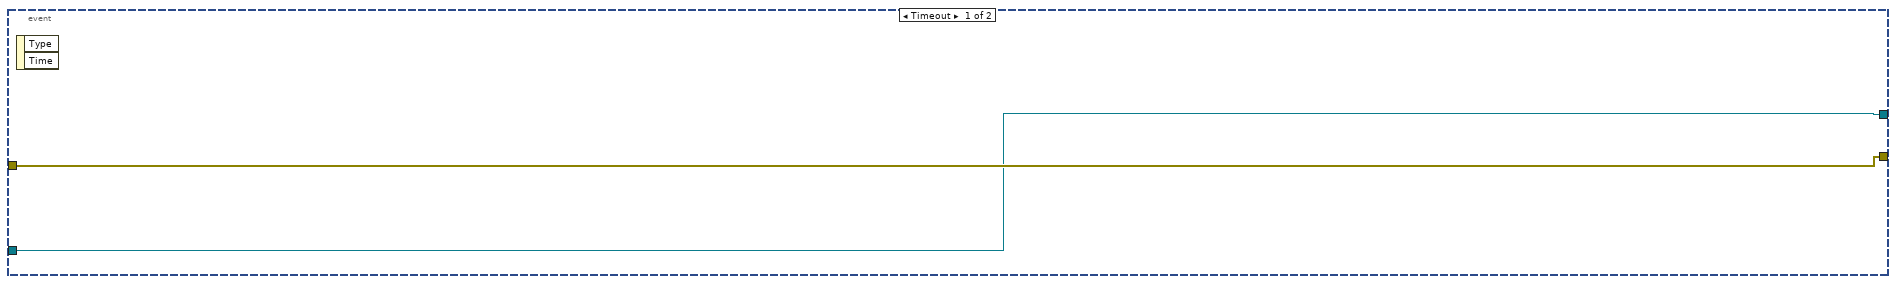
[diagram p12: hidden frame]
diagram:
  n1 = xnode "Open FPGA VI Reference"() -> ("FPGA VI Reference Out"=w12:refnum<k20>, "error out"=w11:errorcluster)  [unwired: 2 in]
  n2 = xnode "Open FPGA VI Reference"() -> ("FPGA VI Reference Out"=w16:refnum<k20>, "error out"=w15:errorcluster)  [unwired: 2 in]
  n3 = while {
    tunnel: w12 -> [w37]
    tunnel: w11 -> [w36]
    tunnel: [w34] -> w6
    tunnel: [w33] -> w5
    stop <- FALSE stop-if-true
    n4 = event shown="[1] \"Internal Setpoint\", \"I scale\", \"P scale\": Value Change" {
      selector: _ -> [_ _]
      dyn-events: _ -> [_ _]
      timeout: _ -> [_ _]
      tunnel: w37 -> [w38 w46]
      tunnel: w36 -> [w39 w45]
      tunnel: [w38 w41] -> w34
      tunnel: [w39 w40] -> w33
      event Timeout {
        n5 = event-data() -> ()  [unwired: 1 in, 2 out]
      }
      event "Internal Setpoint", "I scale", "P scale": Value Change {
        n6 = event-data() -> ()  [unwired: 1 in, 5 out]
        n7 = xnode "Read/Write Control"("FPGA VI Reference In"=w46, "error in"=w45, "Internal Setpoint External Control"="Internal Setpoint", "I scale"="I scale", "P scale"="P scale") -> ("FPGA VI Reference Out"=w41:refnum<k20>, "error out"=w40:errorcluster)
      }
    }
  }
  n8 = while {
    tunnel: w16 -> [w51]
    tunnel: w15 -> [w50]
    tunnel: [w48] -> w2
    tunnel: [w47] -> w1
    stop <- FALSE stop-if-true
    n9 = event shown="[1] \"offset retraction drift\", \" control for drift correction\", \"time before averaging drift\", \"drift averager\", \"drift Waiting (uSec) \", \"offset FM\", \"shift integrator control\", \"upper limit regions\", \"Number of Feedback Regions\": Value Change" {
      selector: _ -> [_ _]
      dyn-events: _ -> [_ _]
      timeout: _ -> [_ _]
      tunnel: w51 -> [w53 w68]
      tunnel: w50 -> [w52 w67]
      tunnel: [w53 w55] -> w48
      tunnel: [w52 w54] -> w47
      event Timeout {
        n10 = event-data() -> ()  [unwired: 1 in, 2 out]
      }
      event "offset retraction drift", "control for drift correction", "time before averaging drift", "drift averager", "drift Waiting (uSec)", "offset FM", "shift integrator control", "upper limit regions", "Number of Feedback Regions": Value Change {
        n11 = event-data() -> ()  [unwired: 1 in, 5 out]
        n12 = Quotient & Remainder(x=u32 65534, y="Number of Feedback Regions") -> (floor(x/y)=w58:u32)  [unwired: 1 out]
        "Steps Per Feedback region" <- w58
        n13 = xnode "Read/Write Control"("FPGA VI Reference In"=w68, "error in"=w67, "offset retraction drift"="offset retraction drift", "drift temporal control"="control for drift correction", "time before averaging drift"="time before averaging drift", "drift averager"="drift averager", "drift Waiting (uSec)"="drift Waiting (uSec)", "offset FM"="offset FM", "Steps per Feedback Region"=w58, "shift integrator control"="shift integrator control", "provisional limit"="upper limit regions", "shift-divisions (always >=2)"="Number of Feedback Regions") -> ("FPGA VI Reference Out"=w55:refnum<k20>, "error out"=w54:errorcluster)
      }
    }
  }
  n14 = xnode "Close FPGA VI Reference"("FPGA VI Reference In"=w2, "error in"=w1) -> ()  [unwired: 1 out]
  n15 = xnode "Close FPGA VI Reference"("FPGA VI Reference In"=w6, "error in"=w5) -> ()  [unwired: 1 out]
  n16 = xnode "Open FPGA VI Reference"() -> ("FPGA VI Reference Out"=w10:refnum<k20>, "error out"=w9:errorcluster)  [unwired: 2 in]
  n17 = xnode "Open FPGA VI Reference"() -> ("FPGA VI Reference Out"=w14:refnum<k20>, "error out"=w13:errorcluster)  [unwired: 2 in]
  n18 = while {
    tunnel: w10 -> [w80]
    tunnel: w9 -> [w79]
    tunnel: [w70] -> w8
    tunnel: [w69] -> w7
    stop <- FALSE stop-if-true
    n19 = xnode "Read/Write Control"("FPGA VI Reference In"=w80, "error in"=w79) -> ("FPGA VI Reference Out"=w70:refnum<k20>, "error out"=w69:errorcluster, "Internal Setpoint"=→"Internal Setpoint indicator":i16, "X Output Value"=→"X Output Value":i16, "Y Output Value"=→"Y Output Value":i16, "Command Out"=→"Command Out":i16, "iterations x"=→"iterations x":i32, "Counter Data"=→"counter":i8, "Inidicator  forth/back  Y axis"=→"Inidicator  forth/back  Y axis":i8)
  }
  n20 = while {
    tunnel: w14 -> [w85]
    tunnel: w13 -> [w84]
    tunnel: [w82] -> w4
    tunnel: [w81] -> w3
    stop <- FALSE stop-if-true
    n21 = event shown="[1] \"Setpoint Control\", \"PID gains (x 2^8)\", \"Forth/Back X axis\", \"Forth/Back Y axis\", \"Stop Feedback\", \"Scanning On/Off\", \"Feedback loop time(uSec)\": Value Change" {
      selector: _ -> [_ _]
      dyn-events: _ -> [_ _]
      timeout: _ -> [_ _]
      tunnel: w85 -> [w87 w98]
      tunnel: w84 -> [w86 w97]
      tunnel: [w87 w89] -> w82
      tunnel: [w86 w88] -> w81
      event Timeout {
        n22 = event-data() -> ()  [unwired: 1 in, 2 out]
      }
      event "Setpoint Control", "PID gains (x 2^8)", "Forth/Back X axis", "Forth/Back Y axis", "Stop Feedback", "Scanning On/Off", "Feedback loop time(uSec)": Value Change {
        n23 = event-data() -> ()  [unwired: 1 in, 5 out]
        n24 = xnode "Read/Write Control"("FPGA VI Reference In"=w98, "error in"=w97, "Setpoint Control"="Setpoint Control", "PID gains (x 2^8)"="PID gains (x 2^8)", "Forth/Back X axis"="Forth/Back X axis", "Forth/Back Y axis"="Forth/Back Y axis", "Count(uSec)"="Feedback loop time(uSec)", "Stop Feedback Control"="Stop Feedback", "Scanning On/Off"="Scanning On/Off") -> ("FPGA VI Reference Out"=w89:refnum<k20>, "error out"=w88:errorcluster)
      }
    }
  }
  n25 = xnode "Open FPGA VI Reference"() -> ("FPGA VI Reference Out"=w22:refnum<k20>, "error out"=w21:errorcluster)  [unwired: 2 in]
  n26 = xnode "Invoke Method"("FPGA VI Reference In"=w22, "error in"=w21) -> ("FPGA VI Reference Out"=w19:refnum<k20>, "error out"=w20:errorcluster)  [unwired: 1 in]
  n27 = xnode "Close FPGA VI Reference"("FPGA VI Reference In"=w4, "error in"=w3) -> ()  [unwired: 1 out]
  n28 = while {
    tunnel: w20 -> [w100]
    tunnel: w19 -> [w103]
    tunnel: [w102] -> w31
    tunnel: [w101] -> w30
    stop <- FALSE stop-if-true
    n29 = event shown="[1] \"X axis pixels\", \"x initial\", \"y initial\", \"Y axis pixels\", \"Timeout FIFO\", \"Time per step/ Y axis sub pixels (usec)\", \"Lines per second\", \"X Size (um)\", \"Y Size (um)\", \"X Total Range (um)\", \"Number of images\", \"Y Total Range (um)\": Value Change" {
      selector: _ -> [_ _]
      dyn-events: _ -> [_ _]
      timeout: _ -> [_ _]
      tunnel: w103 -> [w104 w134]
      tunnel: [w104 w133] -> w102
      tunnel: [w105 w132] -> w101
      tunnel: w100 -> [w105 w131]
      event Timeout {
        n30 = event-data() -> ()  [unwired: 1 in, 2 out]
      }
      event "X axis pixels", "x initial", "y initial", "Y axis pixels", "Timeout FIFO", "Time per step/ Y axis sub pixels (usec)", "Lines per second", "X Size (um)", "Y Size (um)", "X Total Range (um)", "Number of images", "Y Total Range (um)": Value Change {
        # "Number of Y lines"
        # "Time per step Y axis"
        # "Time per step X axis"
        # "Time per pixel x axis"
        # "Image Total Pixels"
        # "Y axis steps per pixel"
        # "Time per pixel / X axis"
        # "X axis steps per pixel"
        n31 = event-data() -> ()  [unwired: 1 in, 5 out]
        n32 = Multiply(x="Y Total Range (um)", y="Y axis pixels") -> (x*y=w139:dbl)
        n33 = Multiply(x="X axis pixels", y="Lines per second") -> (x*y=w151:dbl)
        n34 = Multiply(x="X Total Range (um)", y="X axis pixels") -> (x*y=w145:dbl)
        n35 = Multiply(x="Y Size (um)", y=i16 32767) -> (x*y=w141:dbl)
        n36 = Multiply(x="X Size (um)", y=i16 32767) -> (x*y=w147:dbl)
        n37 = Divide(x=w141, y=w139) -> (x/y=w138:dbl)
        n38 = Divide(x=1.0, y=w151) -> (x/y=w130:dbl)
        n39 = Divide(x=w147, y=w145) -> (x/y=w128:dbl)
        n40 = Multiply(x=w130, y=1000000.0) -> (x*y=w127:dbl)
        n41 = To Unsigned Word Integer(number=w138) -> (unsigned 16bit integer=w123:u16)
        "Y axis steps per pixel" <- w123
        n42 = To Unsigned Word Integer(number=w128) -> (unsigned 16bit integer=w126:u16)
        "X axis steps per pixel" <- w126
        n43 = Quotient & Remainder(x=w127, y=w126) -> (floor(x/y)=w120:dbl)  [unwired: 1 out]
        "Time per step (us) /X axis sub pixels" <- w120
        n44 = To Unsigned Long Integer(number=w127) -> (unsigned 32bit integer=w119:u32)
        n45 = To Unsigned Long Integer(number="Y axis pixels") -> (unsigned 32bit integer=w107:u32)
        n46 = Multiply(x="Y axis pixels", y="Number of images") -> (x*y=w114:u32)
        n47 = Multiply(x="X axis pixels", y=u16 2) -> (x*y=w110:u16)
        n48 = Multiply(x=w107, y=w110) -> (x*y=w109:u32)
        "Pixels for one image" <- w109
        n49 = Multiply(x=w114, y=w110) -> (x*y=w106:u32)
        n50 = Subtract(x=w123, y=u16 1) -> (x-y=w121:u16)
        n51 = Subtract(x=w126, y=u16 1) -> (x-y=w124:u16)
        n52 = Subtract(x=w114, y=u32 1) -> (x-y=w115:u32)
        n53 = Decrement(x="Y axis pixels") -> (x-1=w111:u16)
        n54 = xnode "Read/Write Control"("FPGA VI Reference In"=w134, "error in"=w131, "X axis pixels"="X axis pixels", "x initial"="x initial", "y initial"="y initial", "X steps per pixel"=w124, "Y steps per pixel"=w121, "Y axis pixels"=w111, "Timeout FIFO"="Timeout FIFO", "Time per step/ Y axis sub pixel (uSec)"="Time per step/ Y axis sub pixels (usec)", "Time per image pixel/ X axis pixel (uSec)"=w119, "Time per step/ X axis sub pixel (uSec)"=w120, "Y Number of Lines"=w115, "Image Total Pixels"=w106, "Pixels in one image"=w109) -> ("FPGA VI Reference Out"=w133:refnum<k20>, "error out"=w132:errorcluster)
      }
    }
  }
  n55 = xnode "Close FPGA VI Reference"("FPGA VI Reference In"=w8, "error in"=w7) -> ()  [unwired: 1 out]
  n56 = Generate Occurrence() -> (w24:refnum<k4>)
  n57 = while {
    tunnel: w24 -> [w155]
    shift-right: [w154] -> _
    shift-left: _ -> [w152]
    stop <- FALSE stop-if-true
    n58 = flat-sequence {
      tunnel: w155 -> [w158]
      tunnel: [w157] -> w153
      tunnel: w152 -> [w157]
      tunnel: [w163] -> w154
      tunnel: w153 -> [w161]
      frame #0 {
        n59 = while {
          tunnel: w158 -> [w159]
          stop <- w160 continue-if-true
          n60 = Wait on Occurrence(2:w159) -> (0:w160:bool)  [unwired: 2 in]
        }
      }
      frame #1 {
        w175 = u32[] [0, 65793, 131586, 197379, 263172, 328965, 394758, 460551, 526344, 592137, 657930, 723723, 789516, 855309, 921102, 986895, 1052688, 1118481, 1184274, 1250067, 1315860, 1381653, 1447446, 1513239, 1579032, 1644825, 1710618, 1776411, 1842204, 1907997, 1973790, 2039583, 2105376, 2171169, 2236962, 2302755, 2368548, 2434341, 2500134, 2565927, 2631720, 2697513, 2763306, 2829099, 2894892, 2960685, 3026478, 3092271, 3158064, 3223857, 3289650, 3355443, 3421236, 3487029, 3552822, 3618615, 3684408, 3750201, 3815994, 3881787, 3947580, 4013373, 4079166, 4144959, 4210752, 4276545, 4342338, 4408131, 4473924, 4539717, 4605510, 4671303, 4737096, 4802889, 4868682, 4934475, 5000268, 5066061, 5131854, 5197647, 5263440, 5329233, 5395026, 5460819, 5526612, 5592405, 5658198, 5723991, 5789784, 5855577, 5921370, 5987163, 6052956, 6118749, 6184542, 6250335, 6316128, 6381921, 6447714, 6513507, 6579300, 6645093, 6710886, 6776679, 6842472, 6908265, 6974058, 7039851, 7105644, 7171437, 7237230, 7303023, 7368816, 7434609, 7500402, 7566195, 7631988, 7697781, 7763574, 7829367, 7895160, 7960953, 8026746, 8092539, 8158332, 8224125, 8289918, 8355711, 8421504, 8487297, 8553090, 8618883, 8684676, 8750469, 8816262, 8882055, 8947848, 9013641, 9079434, 9145227, 9211020, 9276813, 9342606, 9408399, 9474192, 9539985, 9605778, 9671571, 9737364, 9803157, 9868950, 9934743, 10000536, 10066329, 10132122, 10197915, 10263708, 10329501, 10395294, 10461087, 10526880, 10592673, 10658466, 10724259, 10790052, 10855845, 10921638, 10987431, 11053224, 11119017, 11184810, 11250603, 11316396, 11382189, 11447982, 11513775, 11579568, 11645361, 11711154, 11776947, 11842740, 11908533, 11974326, 12040119, 12105912, 12171705, 12237498, 12303291, 12369084, 12434877, 12500670, 12566463, 12632256, 12698049, 12763842, 12829635, 12895428, 12961221, 13027014, 13092807, 13158600, 13224393, 13290186, 13355979, 13421772, 13487565, 13553358, 13619151, 13684944, 13750737, 13816530, 13882323, 13948116, 14013909, 14079702, 14145495, 14211288, 14277081, 14342874, 14408667, 14474460, 14540253, 14606046, 14671839, 14737632, 14803425, 14869218, 14935011, 15000804, 15066597, 15132390, 15198183, 15263976, 15329769, 15395562, 15461355, 15527148, 15592941, 15658734, 15724527, 15790320, 15856113, 15921906, 15987699, 16053492, 16119285, 16185078, 16250871, 16316664, 16382457, 16448250, 16514043, 16579836, 16645629, 16711422] ("Array")
        w176 = u32 4417888
        n61 = local read "Trace Topography Array"() -> (w178:i32[][])
        "Trace  Topography" <- w178
        n62 = local read "Topography Array"() -> (→"Topography Image":i32[][])
        n63 = local read "Trace AI2 array"() -> (w179:i16[][])
        "Trace Frequency" <- w179
        n64 = local read "AI2 Array"() -> (→"Frequency Shift Image":i16[][])
        n65 = Array Max & Min(array=w179) -> (max value=w182:i16, min value=w181:i16)  [unwired: 2 out]
        n66 = property on="Frequency Shift Image" class="IntGraph (strict)"("ZScale.Maximum"=w182, "ZScale.Minimum"=w181) -> ()  [unwired: 2 in, 2 out]
        n67 = Array Max & Min(array=w178) -> (max value=w162:i32, min value=w165:i32)  [unwired: 2 out]
        n68 = property on="Topography Image" class="IntGraph (strict)"("ZScale.Maximum"=w162, "ZScale.Minimum"=w165) -> ()  [unwired: 2 in, 2 out]
        n69 = Greater?(x=w162, y=w161) -> (0:w164:bool)
        n70 = local read "Trace AI0 Array"() -> (w177:i16[][])
        "Trace Bottom Sensor Phase" <- w177
        n71 = Select(t=w162, s=w164, f=w161) -> (s? t:f=w163:i32)
        n72 = Array Max & Min(array=w177) -> (max value=w185:i16, min value=w184:i16)  [unwired: 2 out]
        n73 = local read "AI0 Array"() -> (→"Bottom Sensor Phase  Image":i16[][])
        n74 = property on="Topography Image" class="IntGraph (strict)"("Color Table"=w175, "ZScale.Low Color"=w176) -> ()  [unwired: 2 in, 2 out]
        n75 = property on="Bottom Sensor Phase  Image" class="IntGraph (strict)"("ZScale.Maximum"=w185, "ZScale.Minimum"=w184) -> ()  [unwired: 2 in, 2 out]
        n76 = property on="Bottom Sensor Phase  Image" class="IntGraph (strict)"("Color Table"=w175, "ZScale.Low Color"=w176) -> ()  [unwired: 2 in, 2 out]
        n77 = local read "Trace AI6  array"() -> (w172:i16[][])
        "Trace TF Magnitud" <- w172
        n78 = local read "AI6 Array"() -> (→"TF Magnitude Image":i16[][])
        n79 = Array Max & Min(array=w172) -> (max value=w171:i16, min value=w170:i16)  [unwired: 2 out]
        n80 = property on="Frequency Shift Image" class="IntGraph (strict)"("Color Table"=w175, "ZScale.Low Color"=w176) -> ()  [unwired: 2 in, 2 out]
        n81 = property on="TF Magnitude Image" class="IntGraph (strict)"("ZScale.Maximum"=w171, "ZScale.Minimum"=w170) -> ()  [unwired: 2 in, 2 out]
        n82 = local read "Trace AI5 array"() -> (w168:i16[][])
        "Trace Bottom Sensor Magnitude" <- w168
        n83 = local read "AI5 Array"() -> (→"Bottom Sensor Magnitude Image":i16[][])
        n84 = Array Max & Min(array=w168) -> (max value=w167:i16, min value=w166:i16)  [unwired: 2 out]
        n85 = property on="Bottom Sensor Magnitude Image" class="IntGraph (strict)"("ZScale.Maximum"=w167, "ZScale.Minimum"=w166) -> ()  [unwired: 2 in, 2 out]
      }
    }
  }
  n86 = Generate Occurrence() -> (w23:refnum<k4>)
  n87 = xnode "Close FPGA VI Reference"("FPGA VI Reference In"=w31, "error in"=w30) -> ("error out"=→"error out":errorcluster)
  n88 = while {
    tunnel: w23 -> [w186]
    stop <- FALSE stop-if-true
    n89 = case shown="False" "New Image" {
      tunnel: w186 -> [_ w189]
      frame False {
      }
      frame True {
        n90 = Set Occurrence(w189) -> ()
      }
    }
  }
  n91 = xnode "Open FPGA VI Reference"() -> ("FPGA VI Reference Out"=w32:refnum<k20>, "error out"=w26:errorcluster)  [unwired: 2 in]
  n92 = while {
    tunnel: w32 -> [w224]
    tunnel: [w225] -> w29
    tunnel: w26 -> [w223]
    tunnel: [w214] -> w25
    tunnel: w24 -> [w212]
    tunnel: w23 -> [w211]
    shift-right: [w205] -> _
    shift-left: TRUE -> [w201]
    shift-right: [w193] -> _
    shift-left: -1 ("image indicator") -> [w195]
    stop <- FALSE stop-if-true
    n93 = flat-sequence {
      tunnel: [w294] -> w222
      tunnel: [w285] -> w221
      tunnel: [w277] -> w220
      tunnel: [w283] -> w219
      tunnel: [w280] -> w218
      tunnel: [w248] -> w217
      tunnel: [w281] -> w216
      tunnel: [w293] -> w215
      tunnel: [w292] -> w213
      tunnel: w224 -> [w278]
      tunnel: w223 -> [w279]
      tunnel: w212 -> [w292]
      tunnel: [w276] -> w202
      tunnel: w201 -> [w270]
      tunnel: [w245] -> w198
      tunnel: [w253] -> w197
      tunnel: [w251] -> w196
      tunnel: w195 -> [w229]
      tunnel: [w236] -> w194
      tunnel: w222 -> [w324]
      tunnel: w221 -> [w323]
      tunnel: w220 -> [w310]
      tunnel: w219 -> [w322]
      tunnel: w218 -> [w320]
      tunnel: w217 -> [w312]
      tunnel: w216 -> [w318]
      tunnel: w215 -> [w321]
      tunnel: [w324] -> w210
      tunnel: [w321] -> w208
      tunnel: w213 -> [w315]
      tunnel: [w315] -> w206
      tunnel: [w314] -> w203
      tunnel: w202 -> [w314]
      tunnel: [w313] -> w199
      tunnel: w198 -> [w313]
      tunnel: w197 -> [w311]
      tunnel: w196 -> [w309]
      tunnel: w194 -> [w308]
      tunnel: [w308] -> w191
      tunnel: w210 -> [w385]
      tunnel: [w385] -> w209
      tunnel: w208 -> [w384]
      tunnel: [w384] -> w207
      tunnel: w206 -> [w380]
      tunnel: [w383] -> w204
      tunnel: w203 -> [w383]
      tunnel: [w382] -> w200
      tunnel: w199 -> [w382]
      tunnel: [w381] -> w192
      tunnel: w191 -> [w381]
      tunnel: [w380] -> w190
      tunnel: [w391] -> w214
      tunnel: [w392] -> w225
      tunnel: w209 -> [w392]
      tunnel: w207 -> [w391]
      tunnel: w211 -> [w390]
      tunnel: [w389] -> w205
      tunnel: w204 -> [w389]
      tunnel: w200 -> [w388]
      tunnel: [w387] -> w193
      tunnel: w192 -> [w387]
      tunnel: w190 -> [w386]
      frame #0 {
        # "1024 is just a number\nlarger than 512 but less\nthan total pixel images"
        n94 = local read "X axis pixels"() -> (w267:u16)
        n95 = xnode "Invoke Method"("FPGA VI Reference In"=w278, "error in"=w279, "Number of Elements"=w267, "Timeout (ms)"=-1) -> ("FPGA VI Reference Out"=w291:refnum<k20>, "error out"=w290:errorcluster, "Data"=w266:u64[])  [unwired: 1 out]
        n96 = Decimate 1D Array(w266) -> (w265:u64[], w262:u64[])
        n97 = local read "Pixels for one image"() -> (w273:i32)
        n98 = To Unsigned Long Integer(number=w262) -> (unsigned 32bit integer=w261:u32[])
        n99 = Split Number(x=w265) -> (hi(x)=w303:u32[], lo(x)=w302:u32[])
        n100 = Split Number(x=w261) -> (hi(x)=w258:u16[], lo(x)=w255:u16[])
        n101 = xnode "Read/Write Control"("FPGA VI Reference In"=w291, "error in"=w290) -> ("FPGA VI Reference Out"=w288:refnum<k20>, "error out"=w289:errorcluster, "Indicator  forth/back X axis"=w248:i8, "iterations x"=w272:i32, "Y line"=w233:i32)
        "Y line" <- w233
        n102 = Less Or Equal?(x=w272, y=w267) -> (x <= y?=w271:bool)
        n103 = Split Number(x=w303) -> (hi(x)=w301:u16[], lo(x)=w235:u16[])
        "hi(x)" <- w235
        n104 = Split Number(x=w302) -> (hi(x)=w298:u16[], lo(x)=w296:u16[])
        n105 = local read "Y axis pixels"() -> (w232:u16)
        n106 = Select(t=TRUE, s=w271, f=w270) -> (s? t:f=w269:bool)
        n107 = First Call?() -> (First Call?: T/F=w234:bool)
        n108 = Increment(x=w272) -> (x+1=w275:i32)
        n109 = xnode "Invoke Method"("FPGA VI Reference In"=w288, "error in"=w289, "Number of Elements"=w267, "Timeout (ms)"=-1) -> ("FPGA VI Reference Out"=w294:refnum<k20>, "error out"=w293:errorcluster, "Data"=w264:u64[])  [unwired: 1 out]
        n110 = Quotient & Remainder(x=w275, y=w273) -> (x-y*floor(x/y)=w243:i32)  [unwired: 1 out]
        n111 = Less Or Equal?(x=w243, y=w267) -> (x <= y?=w240:bool)
        n112 = Decrement(x=w232) -> (x-1=w227:u16)
        n113 = Quotient & Remainder(x=w233, y=w227) -> (floor(x/y)=w231:i32)  [unwired: 1 out]
        "fpga y images" <- w231
        n114 = Add(x=w231, y=w229) -> (x+y=w230:i32)
        n115 = Select(t=w230, s=w234, f=w229) -> (s? t:f=w228:i32)
        n116 = Increment(x=w228) -> (x+1=w239:i32)
        n117 = Select(t=w239, s=w240, f=w228) -> (s? t:f=w236:i32)
        "line shift" <- w236
        n118 = Increment(x=w236) -> (x+1=→"image indicator":i32)
        n119 = Add(x=w233, y=w236) -> (x+y=w237:i32)
        n120 = Quotient & Remainder(x=w237, y=w232) -> (x-y*floor(x/y)=w244:i32)  [unwired: 1 out]
        n121 = Decimate 1D Array(w264) -> (w263:u64[], w260:u64[])
        n122 = Not(x=w269) -> (.not. x?=w274:bool)
        n123 = To Unsigned Long Integer(number=w260) -> (unsigned 32bit integer=w259:u32[])
        n124 = Select(t=w274, s=w240, f=w269) -> (s? t:f=w276:bool)
        n125 = Split Number(x=w259) -> (hi(x)=w257:u16[], lo(x)=w256:u16[])
        n126 = Split Number(x=w263) -> (hi(x)=w307:u32[], lo(x)=w306:u32[])
        n127 = Split Number(x=w307) -> (hi(x)=w300:u16[], lo(x)=w299:u16[])
        n128 = Split Number(x=w306) -> (hi(x)=w297:u16[], lo(x)=w295:u16[])
        n129 = Equal?(x=w248, y=i8 -1) -> (x = y?=w246:bool)
        n130 = Subtract(x=w227, y=w244) -> (x-y=w287:i32)
        n131 = Equal?(x=w244, y=255) -> (x = y?=w250:bool)
        n132 = Greater?(x=w243, y=1024) -> (0:w241:bool)
        n133 = Select(t=w244, s=w276, f=w287) -> (s? t:f=w277:i32)
        "line in matrix" <- w277
        n134 = Compound Arithmetic op=AND(w241, w250, w246) -> (w245:bool)
        n135 = Build Array (concatenate)(w258, w257) -> (w254:u16[])
        n136 = Build Array (concatenate)(w255, w256) -> (w252:u16[])
        n137 = Build Array (concatenate)(w298, w297) -> (w280:u16[])
        n138 = Build Array (concatenate)(w296, w295) -> (w282:u16[])
        n139 = Build Array (concatenate)(w235, w299) -> (w284:u16[])
        n140 = Build Array (concatenate)(w301, w300) -> (w286:u16[])
        n141 = To Word Integer(number=w254) -> (16bit integer=w253:i16[])
        n142 = To Word Integer(number=w252) -> (16bit integer=w251:i16[])
        n143 = To Word Integer(number=w284) -> (16bit integer=w283:i16[])
        n144 = To Word Integer(number=w286) -> (16bit integer=w285:i16[])
        n145 = To Word Integer(number=w282) -> (16bit integer=w281:i16[])
      }
      frame #1 {
        n146 = Multiply(x=w320, y=65535) -> (x*y=w317:i32[])
        n147 = Add(x=w317, y=w318) -> (x+y=w316:i32[])
        n148 = case shown="-1" w312 {
          tunnel: w316 -> [w347 w357]
          tunnel: w310 -> [w349 w354]
          frame 1, Default {
            n149 = local read "Topography Array"() -> (w350:i32[][])
            n150 = Replace Array Subset(array=w350, new element=w347, index (col)=w349) -> (w348:i32[][])  [unwired: 1 in]
            n151 = local write "Topography Array"(w348) -> ()
            "Trace Topography Array temp" <- w347
          }
          frame -1 {
            n152 = local read "Trace Topography Array temp"() -> (w351:i32[])
            n153 = Reverse 1D Array(array=w357) -> (reversed array=w353:i32[])
            n154 = local read "Topography Array back"() -> (w355:i32[][])
            n155 = Build Array(w351, w353) -> (→"Trace Topography Array":i32[][])
            n156 = Replace Array Subset "Replace Array Subset"(array=w355, new element=w353, index (col)=w354) -> (w356:i32[][])  [unwired: 1 in]
            n157 = local write "Topography Array back"(w356) -> ()
          }
        }
        n158 = case shown="-1" w312 {
          tunnel: w311 -> [w342 w346]
          tunnel: w310 -> [w341 w344]
          frame -1 {
            n159 = local read "AI6 Array Back"() -> (w340:i16[][])
            n160 = Reverse 1D Array(array=w342) -> (reversed array=w337:i16[])
            n161 = local read "TraceAI6 temp"() -> (w338:i16[])
            n162 = Replace Array Subset(array=w340, new element=w337, index (col)=w341) -> (w339:i16[][])  [unwired: 1 in]
            n163 = local write "AI6 Array Back"(w339) -> ()
            n164 = Build Array(w338, w337) -> (→"Trace AI6  array":i16[][])
          }
          frame 1, Default {
            n165 = local read "AI6 Array"() -> (w345:i16[][])
            n166 = Replace Array Subset(array=w345, new element=w346, index (col)=w344) -> (w343:i16[][])  [unwired: 1 in]
            n167 = local write "AI6 Array"(w343) -> ()
            "TraceAI6 temp" <- w346
          }
        }
        n168 = case shown="-1" w312 {
          tunnel: w322 -> [w358 w368]
          tunnel: w310 -> [w359 w365]
          frame 1, Default {
            n169 = local read "AI2 Array"() -> (w361:i16[][])
            n170 = Replace Array Subset(array=w361, new element=w358, index (col)=w359) -> (w360:i16[][])  [unwired: 1 in]
            n171 = local write "AI2 Array"(w360) -> ()
            "TraceAI2 array temp" <- w358
          }
          frame -1 {
            n172 = local read "TraceAI2 array temp"() -> (w362:i16[])
            n173 = Reverse 1D Array(array=w368) -> (reversed array=w363:i16[])
            n174 = local read "AI2 Array back"() -> (w367:i16[][])
            n175 = Replace Array Subset(array=w367, new element=w363, index (col)=w365) -> (w366:i16[][])  [unwired: 1 in]
            n176 = Build Array(w362, w363) -> (→"Trace AI2 array":i16[][])
            n177 = local write "AI2 Array back"(w366) -> ()
          }
        }
        n178 = case shown="-1" w312 {
          tunnel: w323 -> [w369 w379]
          tunnel: w310 -> [w372 w376]
          frame 1, Default {
            n179 = local read "AI0 Array"() -> (w371:i16[][])
            n180 = Replace Array Subset(array=w371, new element=w369, index (col)=w372) -> (w370:i16[][])  [unwired: 1 in]
            n181 = local write "AI0 Array"(w370) -> ()
            "Trace AI0 array temp" <- w369
          }
          frame -1 {
            n182 = local read "Trace AI0 array temp"() -> (w375:i16[])
            n183 = Reverse 1D Array(array=w379) -> (reversed array=w374:i16[])
            n184 = local read "AI0 back"() -> (w378:i16[][])
            n185 = Replace Array Subset(array=w378, new element=w374, index (col)=w376) -> (w377:i16[][])  [unwired: 1 in]
            n186 = Build Array(w375, w374) -> (→"Trace AI0 Array":i16[][])
            n187 = local write "AI0 back"(w377) -> ()
          }
        }
        n188 = case shown="-1" w312 {
          tunnel: w310 -> [w329 w335]
          tunnel: w309 -> [w331 w332]
          frame -1 {
            n189 = local read "AI5 Back"() -> (w330:i16[][])
            n190 = Reverse 1D Array(array=w331) -> (reversed array=w327:i16[])
            n191 = local read "Trace AI5 temp"() -> (w326:i16[])
            n192 = Replace Array Subset(array=w330, new element=w327, index (col)=w329) -> (w328:i16[][])  [unwired: 1 in]
            n193 = local write "AI5 Back"(w328) -> ()
            n194 = Build Array(w326, w327) -> (→"Trace AI5 array":i16[][])
          }
          frame 1, Default {
            n195 = local read "AI5 Array"() -> (w334:i16[][])
            n196 = Replace Array Subset(array=w334, new element=w332, index (col)=w335) -> (w333:i16[][])  [unwired: 1 in]
            n197 = local write "AI5 Array"(w333) -> ()
            "Trace AI5 temp" <- w332
          }
        }
      }
      frame #2 {
        n198 = Set Occurrence(w380) -> ()
      }
      frame #3 {
        n199 = case shown="True" w388 {
          tunnel: w390 -> [_ w395]
          tunnel: w386 -> [_ w394]
          frame False {
          }
          frame True {
            n200 = flat-sequence {
              tunnel: w395 -> [w397]
              tunnel: w394 -> [w396]
              tunnel: [w396] -> w393
              tunnel: w393 -> [w398]
              frame #0 {
                n201 = Set Occurrence(w397) -> ()
              }
              frame #1 {
                n202 = while {
                  tunnel: w398 -> [w399]
                  stop <- w400 continue-if-true
                  n203 = Wait on Occurrence(2:w399) -> (0:w400:bool)  [unwired: 2 in]
                }
              }
            }
          }
        }
      }
    }
  }
  n204 = while {
    tunnel: w23 -> [w405]
    tunnel: w24 -> [w401]
    stop <- FALSE stop-if-true
    n205 = flat-sequence {
      tunnel: [w415] -> w404
      tunnel: w405 -> [w415]
      tunnel: [w414] -> w402
      tunnel: w401 -> [w414]
      tunnel: w404 -> [w420]
      tunnel: [w420] -> w403
      tunnel: w402 -> [w419]
      tunnel: w403 -> [w421]
      frame #0 {
        w407 = i16 0 ("element")
        w413 = i16 0 ("element")
        n206 = local read "Y axis pixels"() -> (w411:u16)
        n207 = local read "X axis pixels"() -> (w412:u16)
        n208 = Initialize Array(0 ("element"), w411, w412) -> (→"Topography Array" →"Topography Array back":i32[][])
        n209 = Initialize Array(w407, w411, w412) -> (→"AI6 Array" →"AI6 Array Back":i16[][])
        n210 = Initialize Array(w407, w411, w412) -> (→"AI0 Array" →"AI0 back":i16[][])
        n211 = Initialize Array(w413, w411, w412) -> (→"AI2 Array" →"AI2 Array back":i16[][])
        n212 = Initialize Array(w413, w411, w412) -> (→"AI5 Array" →"AI5 Back":i16[][])
      }
      frame #1 {
        n213 = Set Occurrence(w419) -> ()
      }
      frame #2 {
        n214 = while {
          tunnel: w421 -> [w422]
          stop <- w423 continue-if-true
          n215 = Wait on Occurrence(2:w422) -> (0:w423:bool)  [unwired: 2 in]
        }
      }
      frame #3 {
        w430 = TRUE ("transpose? (no:F)")
        w431 = "," ("delimiter (\\t)")
        w438 = ".csv" ("string")
        w439 = "-rev" ("string")
        w436 = "%.6f" ("format (%.3f)")
        w448 = ".csv" ("string")
        w462 = "%.6f" ("format (%.3f)")
        n216 = Get Date/Time In Seconds() -> (seconds since 1Jan1904=w488:timestamp)
        n217 = Format Date/Time String(time format string (%c)="%Y-%m-%d-%H-%M-%S", seconds (now)=w488) -> (date/time string=w425:string)  [unwired: 1 in]
        n218 = Concatenate Strings(w425, "Freq Prefix 1", "Freq Prefix 2", "AI2" ("string")) -> (w451:string)
        n219 = Concatenate Strings(w451, ".csv" ("string")) -> (w485:string)
        n220 = Concatenate Strings(w425, "Phase Prefix 1", "Phase Prefix 2", "AI0" ("string")) -> (w453:string)
        n221 = Concatenate Strings(w425, "Topo Prefix 1", "Topo Prefix 2", "Topography" ("string")) -> (w457:string)
        n222 = Concatenate Strings(w457, ".csv" ("string")) -> (w474:string)
        n223 = Concatenate Strings(w453, ".csv" ("string")) -> (w475:string)
        n224 = local read "AI5 Array"() -> (w435:i16[][])
        n225 = local read "AI6 Array"() -> (w434:i16[][])
        n226 = Build Path(base path="Data Directory", name or relative path=w475) -> (appended path=w473:path)
        n227 = Build Path(base path="Data Directory", name or relative path=w474) -> (appended path=w472:path)
        n228 = Build Path(base path="Data Directory", name or relative path=w485) -> (appended path=w484:path)
        n229 = local read "Topography Array"() -> (w471:i32[][])
        n230 = local read "AI0 Array"() -> (w470:i16[][])
        n231 = local read "AI2 Array"() -> (w491:i16[][])
        n232 = Concatenate Strings(w425, "AI6" ("string")) -> (w437:string)
        n233 = Concatenate Strings(w425, "AI5" ("string")) -> (w445:string)
        n234 = Concatenate Strings(w437, w448) -> (w447:string)
        n235 = Concatenate Strings(w445, w448) -> (w450:string)
        n236 = Build Path(base path="Data Directory", name or relative path=w450) -> (appended path=w449:path)
        n237 = call-poly <vilib>:"Write To Spreadsheet File.vi"("delimiter (\\t)"=w431, "transpose? (no:F)"=w430, "format (%d)"="%.6f" ("format (%.3f)"), "2D data"=w471, "file path (dialog if empty)"=w472) -> ()  [unwired: 3 in, 1 out]
        n238 = Build Path(base path="Data Directory", name or relative path=w447) -> (appended path=w446:path)
        n239 = call-poly <vilib>:"Write To Spreadsheet File.vi"("delimiter (\\t)"=w431, "transpose? (no:F)"=w430, "format (%d)"="%.6f" ("format (%.3f)"), "2D data"=w470, "file path (dialog if empty)"=w473) -> ()  [unwired: 3 in, 1 out]
        n240 = call-poly <vilib>:"Write To Spreadsheet File.vi"("delimiter (\\t)"=w431, "transpose? (no:F)"=w430, "format (%d)"=w462, "2D data"=w491, "file path (dialog if empty)"=w484) -> ()  [unwired: 3 in, 1 out]
        n241 = call-poly <vilib>:"Write To Spreadsheet File.vi"("delimiter (\\t)"=w431, "transpose? (no:F)"=w430, "format (%d)"=w436, "2D data"=w434, "file path (dialog if empty)"=w446) -> ()  [unwired: 3 in, 1 out]
        n242 = call-poly <vilib>:"Write To Spreadsheet File.vi"("delimiter (\\t)"=w431, "transpose? (no:F)"=w430, "format (%d)"=w436, "2D data"=w435, "file path (dialog if empty)"=w449) -> ()  [unwired: 3 in, 1 out]
        n243 = Concatenate Strings(w451, "-rev" ("string"), ".csv" ("string")) -> (w467:string)
        n244 = local read "AI2 Array back"() -> (w452:i16[][])
        n245 = Concatenate Strings(w453, "-rev" ("string"), ".csv" ("string")) -> (w455:string)
        n246 = Concatenate Strings(w457, "-rev" ("string"), ".csv" ("string")) -> (w458:string)
        n247 = local read "Topography Array back"() -> (w461:i32[][])
        n248 = local read "AI0 back"() -> (w460:i16[][])
        n249 = Build Path(base path="Data Directory", name or relative path=w455) -> (appended path=w454:path)
        n250 = Build Path(base path="Data Directory", name or relative path=w467) -> (appended path=w459:path)
        n251 = local read "AI5 Back"() -> (w433:i16[][])
        n252 = local read "AI6 Array Back"() -> (w432:i16[][])
        n253 = Build Path(base path="Data Directory", name or relative path=w458) -> (appended path=w456:path)
        n254 = call-poly <vilib>:"Write To Spreadsheet File.vi"("delimiter (\\t)"=w431, "transpose? (no:F)"=w430, "format (%d)"=w462, "2D data"=w452, "file path (dialog if empty)"=w459) -> ()  [unwired: 3 in, 1 out]
        n255 = call-poly <vilib>:"Write To Spreadsheet File.vi"("delimiter (\\t)"=w431, "transpose? (no:F)"=w430, "format (%d)"=w462, "2D data"=w460, "file path (dialog if empty)"=w454) -> ()  [unwired: 3 in, 1 out]
        n256 = call-poly <vilib>:"Write To Spreadsheet File.vi"("delimiter (\\t)"=w431, "transpose? (no:F)"=w430, "format (%d)"=w462, "2D data"=w461, "file path (dialog if empty)"=w456) -> ()  [unwired: 3 in, 1 out]
        n257 = Concatenate Strings(w445, w439, w438) -> (w444:string)
        n258 = Concatenate Strings(w437, w439, w438) -> (w441:string)
        n259 = Build Path(base path="Data Directory", name or relative path=w444) -> (appended path=w443:path)
        n260 = Build Path(base path="Data Directory", name or relative path=w441) -> (appended path=w442:path)
        n261 = call-poly <vilib>:"Write To Spreadsheet File.vi"("delimiter (\\t)"=w431, "transpose? (no:F)"=w430, "format (%d)"=w436, "2D data"=w432, "file path (dialog if empty)"=w442) -> ()  [unwired: 3 in, 1 out]
        n262 = call-poly <vilib>:"Write To Spreadsheet File.vi"("delimiter (\\t)"=w431, "transpose? (no:F)"=w430, "format (%d)"=w436, "2D data"=w433, "file path (dialog if empty)"=w443) -> ()  [unwired: 3 in, 1 out]
      }
    }
  }
  n263 = xnode "Close FPGA VI Reference"("FPGA VI Reference In"=w29, "error in"=w25) -> ("error out"=→"error out 2":errorcluster)
